vi "I-V measurement.vi"(5 "Session properties":T4, 7 "Workspace":path, 8 "Error In":errorcluster, 9 "myDLTS file path":path=path "", 10 "IV measurement":T1={"Name"="", "Comment"="", "Time"=timestamp(0 s since 1904-01-01), "Folder"=path "", "IV properties"={"T"=0.0, "Vstart"=-0.5, "Vstop"=0.5, "Vpoints"=10.0, "Settling"=0.01, "I limit"=0.1, "Log mapping"=FALSE, "Averaging"=0.0}, "GUID"=""} {"IV properties"."Settling" min=0.0 max=65535.0}, 11 "Loop data":T5={"Persistent"={"Last file"=path "", "Last user"="", "Users"=[]}, "Temp handle"={"Connected"=FALSE, "Temp ctrl"={"Gain (P)"=0.0, "Reset (I)"=0.0, "Rate (D)"=0.0, "Stabilization rate"=0.0, "Stabilization delta"=0.0, "Type"=enum."Lake Shore 325", "Custom temp ctrl"={"VISA resource name"=""}, "Lakeshore 325"={"VISA name"="", "Loop"=0, "Heater Range"=1, "Heater Resistance"=0, "Sample sensor"=0, "Fast sensor"=0, "Slow sensor"=0}, "Lakeshore 331"={"VISA name"="", "Loop"=1, "Heater Range"=0, "Sample sensor"=0, "Fast sensor"=0, "Slow sensor"=0}, "Lakeshore 332"={"VISA name"="", "Loop"=1, "Heater Range"=0, "Sample sensor"=0, "Fast sensor"=0, "Slow sensor"=0}, "Lakeshore 335"={"VISA name"="", "Loop"=1, "Sample sensor"=0, "Fast sensor"=0, "Slow sensor"=0, "Heater Range"=0, "Output mode"=enum."Off"}, "Lakeshore 336"={"VISA name"="", "Loop"=1, "Output mode"=enum."Off", "Max current"=1.0, "Heater resistance"=1, "Sample sensor"=1, "Slow sensor"=1, "Fast sensor"=1}}}, "Paths"={"Manual"=path "", "Settings"=path "", "Persistent"=path "", "Work dir."=path ""}, "Settings"={"MFIA"={"Address"="", "Use compensation"=TRUE, "Shut down gracefully"=FALSE}, "Temp ctrl"={"Gain (P)"=0.0, "Reset (I)"=0.0, "Rate (D)"=0.0, "Stabilization rate"=0.0, "Stabilization delta"=0.0, "Type"=enum."Lake Shore 325", "Custom temp ctrl"={"VISA resource name"=""}, "Lakeshore 325"={"VISA name"="", "Loop"=0, "Heater Range"=1, "Heater Resistance"=0, "Sample sensor"=0, "Fast sensor"=0, "Slow sensor"=0}, "Lakeshore 331"={"VISA name"="", "Loop"=1, "Heater Range"=0, "Sample sensor"=0, "Fast sensor"=0, "Slow sensor"=0}, "Lakeshore 332"={"VISA name"="", "Loop"=1, "Heater Range"=0, "Sample sensor"=0, "Fast sensor"=0, "Slow sensor"=0}, "Lakeshore 335"={"VISA name"="", "Loop"=1, "Sample sensor"=0, "Fast sensor"=0, "Slow sensor"=0, "Heater Range"=0, "Output mode"=enum."Off"}, "Lakeshore 336"={"VISA name"="", "Loop"=1, "Output mode"=enum."Off", "Max current"=1.0, "Heater resistance"=1, "Sample sensor"=1, "Slow sensor"=1, "Fast sensor"=1}}, "Source-meter"={"Type"=enum."Custom", "Custom source-meter"={"VISA resource name"=""}, "Keithley 2600"={"VISA name"="", "Ignore ID Query"=FALSE, "SMU"=enum."Channel A"}, "Keithley 2400 Series"={"VISA name"="", "Ignore ID Query"=FALSE}}, "Other"={"Enable OriginLab"=FALSE, "Reader mode"=FALSE, "Auto-save"=FALSE}, "Defaults"={"IV properties"={"T"=0.0, "Vstart"=-0.5, "Vstop"=0.5, "Vpoints"=10.0, "Settling"=0.01, "I limit"=0.1, "Log mapping"=FALSE, "Averaging"=0.0}, "CV properties"={"T"=0.0, "Vstart"=-0.5, "Vstop"=0.5, "Vpoints"=10.0, "Precision"=enum."Normal", "Test signal"=0.01, "Auto I range"=FALSE, "Test frequency"=100000.0, "I range"=-2.0, "V range"=10.0, "Log mapping"=FALSE, "Rel perm"=0.0, "Area"=0.0, "Equivalent circuit model"=0}, "DLTS properties"={"Tstart"=0.0, "Instant start"=FALSE, "Tstop"=0.0, "T rate"=0.0, "Test signal"=0.0, "Test frequency"=0.0, "Bandwidth"=0.0, "Averaging"=0.0, "Vbias"=0.0, "Vpulse"=0.0, "pulse length"=0.0, "Pulse 2"=FALSE, "Vpulse 2"=0.0, "pulse length 2"=0.0, "I range"=-2.0, "V range"=10.0, "Emission rate"=[], "Sampling rate"=0.0, "Acq. delay"=0.0, "Filter order"=0, "Equivalent circuit model"=0}, "LDLTS properties"={"T"=0.0, "Test signal"=0.0, "Test frequency"=0.0, "Bandwidth"=0.0, "Averaging"=0.0, "Vbias"=0.0, "Vpulse"=0.0, "pulse length"=0.0, "Pulse 2"=FALSE, "Vpulse 2"=0.0, "pulse length 2"=0.0, "I range"=-2.0, "V range"=10.0, "Sampling rate"=0.0, "Acq. delay"=0.0, "Sampling time"=0.0, "Filter order"=0, "Equivalent circuit model"=0}}}, "Software version"=0.0, "MFIA handle"={"ziHandle"={"handleValid"=FALSE, "Conn"=0, "Path Prefix"="", "Handle"=0, "Connected"=FALSE, "Clockbase(s)"=0.0}, "Selected device"="", "ziModHandle"={"handleValid"=FALSE, "Conn"=0, "ModHandle"=0, "moduleID"="", "Path Prefix"=""}}, "Source-meter handle"={"Connected"=FALSE, "Source-meter"={"Type"=enum."Custom", "Custom source-meter"={"VISA resource name"=""}, "Keithley 2600"={"VISA name"="", "Ignore ID Query"=FALSE, "SMU"=enum."Channel A"}, "Keithley 2400 Series"={"VISA name"="", "Ignore ID Query"=FALSE}}}} {"MFIA handle"."ziModHandle"."ModHandle" format="0x%08x"; "MFIA handle"."ziModHandle"."Conn" format="0x%08x"; "MFIA handle"."ziHandle"."Handle" format="0x%08x"; "MFIA handle"."ziHandle"."Conn" format="0x%08x"; "Settings"."Defaults"."LDLTS properties"."Equivalent circuit model" items=["Rp || Cp", "Rs + Cs", "Rs + Ls", "G B", "D Cs", "Q Cs", "D Ls", "Q Ls", "Rp || Lp", "D Cp"]; "Settings"."Defaults"."LDLTS properties"."Filter order" min=0 max=8 step=1; "Settings"."Defaults"."LDLTS properties"."Sampling rate" items=["13k"=13392.857422, "27k"=26785.714844, "54k"=53571.429687, "107k"=107142.859375]; "Settings"."Defaults"."LDLTS properties"."V range" items=["10mV"=0.01, "100mV"=0.1, "1V"=1.0, "10V"=10.0]; "Settings"."Defaults"."LDLTS properties"."I range" items=["100nA"=-7.0, "1µA"=-6.0, "10µA"=-5.0, "100µA"=-4.0, "1mA"=-3.0, "10mA"=-2.0]; "Settings"."Defaults"."DLTS properties"."Equivalent circuit model" items=["Rp || Cp", "Rs + Cs", "Rs + Ls", "G B", "D Cs", "Q Cs", "D Ls", "Q Ls", "Rp || Lp", "D Cp"]; "Settings"."Defaults"."DLTS properties"."Filter order" min=0 max=8 step=1; "Settings"."Defaults"."DLTS properties"."Sampling rate" items=["13k"=13392.857422, "27k"=26785.714844, "54k"=53571.429687, "107k"=107142.859375]; "Settings"."Defaults"."DLTS properties"."V range" items=["10mV"=0.01, "100mV"=0.1, "1V"=1.0, "10V"=10.0]; "Settings"."Defaults"."DLTS properties"."I range" items=["10mV"=0.01, "100mV"=0.1, "1V"=1.0, "10V"=10.0]; "Settings"."Defaults"."CV properties"."Equivalent circuit model" items=["Rp || Cp", "Rs + Cs", "Rs + Ls", "G B", "D Cs", "Q Cs", "D Ls", "Q Ls", "Rp || Lp", "D Cp"]; "Settings"."Defaults"."CV properties"."V range" items=["10mV"=0.01, "100mV"=0.1, "1V"=1.0, "10V"=10.0]; "Settings"."Defaults"."CV properties"."I range" items=["100nA"=-7.0, "1µA"=-6.0, "10µA"=-5.0, "100µA"=-4.0, "1mA"=-3.0, "10mA"=-2.0]; "Settings"."Defaults"."IV properties"."Settling" min=0.0 max=65535.0; "Settings"."Temp ctrl"."Lakeshore 336"."Fast sensor" items=["Sensor A", "Sensor B", "Sensor C", "Sensor D"]; "Settings"."Temp ctrl"."Lakeshore 336"."Slow sensor" items=["Sensor A", "Sensor B", "Sensor C", "Sensor D"]; "Settings"."Temp ctrl"."Lakeshore 336"."Sample sensor" items=["Sensor A", "Sensor B", "Sensor C", "Sensor D"]; "Settings"."Temp ctrl"."Lakeshore 336"."Heater resistance" items=["25 Ohm"=1, "50 Ohm"=2]; "Settings"."Temp ctrl"."Lakeshore 336"."Max current" items=["0.707 A"=0.0, "1 A"=1.0, "1.414 A"=1.414, "2 A"=2.0]; "Settings"."Temp ctrl"."Lakeshore 336"."Loop" items=["Output 1"=1, "Output 2"=2, "Output 3"=3, "Output 4"=4]; "Settings"."Temp ctrl"."Lakeshore 335"."Heater Range" items=["Off", "Low (On)", "Medium", "High"]; "Settings"."Temp ctrl"."Lakeshore 335"."Slow sensor" items=["A", "B"]; "Settings"."Temp ctrl"."Lakeshore 335"."Fast sensor" items=["A", "B"]; "Settings"."Temp ctrl"."Lakeshore 335"."Sample sensor" items=["A", "B"]; "Settings"."Temp ctrl"."Lakeshore 335"."Loop" items=["Loop 1"=1, "Loop 2"=2]; "Settings"."Temp ctrl"."Lakeshore 332"."Slow sensor" items=["A", "B"]; "Settings"."Temp ctrl"."Lakeshore 332"."Fast sensor" items=["A", "B"]; "Settings"."Temp ctrl"."Lakeshore 332"."Sample sensor" items=["A", "B"]; "Settings"."Temp ctrl"."Lakeshore 332"."Heater Range" items=["Off", "Low (0.5W)", "Med (5W)", "High (50W)"]; "Settings"."Temp ctrl"."Lakeshore 332"."Loop" items=["Loop 1", "Loop 2"]; "Settings"."Temp ctrl"."Lakeshore 331"."Slow sensor" items=["A", "B"]; "Settings"."Temp ctrl"."Lakeshore 331"."Fast sensor" items=["A", "B"]; "Settings"."Temp ctrl"."Lakeshore 331"."Sample sensor" items=["A", "B"]; "Settings"."Temp ctrl"."Lakeshore 331"."Heater Range" items=["Off", "Low (0.5W)", "Med (5W)", "High (50W)"]; "Settings"."Temp ctrl"."Lakeshore 331"."Loop" items=["Loop 1", "Loop 2"]; "Settings"."Temp ctrl"."Lakeshore 325"."Slow sensor" items=["A", "B"]; "Settings"."Temp ctrl"."Lakeshore 325"."Fast sensor" items=["A", "B"]; "Settings"."Temp ctrl"."Lakeshore 325"."Sample sensor" items=["A", "B"]; "Settings"."Temp ctrl"."Lakeshore 325"."Heater Resistance" items=["25 Ohm"=1, "50 Ohm"=2]; "Settings"."Temp ctrl"."Lakeshore 325"."Heater Range" items=["Off", "Low (loop 1) or On (loop 2)", "High (loop 1)"]; "Settings"."Temp ctrl"."Lakeshore 325"."Loop" items=["Loop 1"=1, "Loop 2"=2]; "Temp handle"."Temp ctrl"."Lakeshore 336"."Fast sensor" items=["Sensor A", "Sensor B", "Sensor C", "Sensor D"]; "Temp handle"."Temp ctrl"."Lakeshore 336"."Slow sensor" items=["Sensor A", "Sensor B", "Sensor C", "Sensor D"]; "Temp handle"."Temp ctrl"."Lakeshore 336"."Sample sensor" items=["Sensor A", "Sensor B", "Sensor C", "Sensor D"]; "Temp handle"."Temp ctrl"."Lakeshore 336"."Heater resistance" items=["25 Ohm"=1, "50 Ohm"=2]; "Temp handle"."Temp ctrl"."Lakeshore 336"."Max current" items=["0.707 A"=0.0, "1 A"=1.0, "1.414 A"=1.414, "2 A"=2.0]; "Temp handle"."Temp ctrl"."Lakeshore 336"."Loop" items=["Output 1"=1, "Output 2"=2, "Output 3"=3, "Output 4"=4]; "Temp handle"."Temp ctrl"."Lakeshore 335"."Heater Range" items=["Off", "Low (On)", "Medium", "High"]; "Temp handle"."Temp ctrl"."Lakeshore 335"."Slow sensor" items=["A", "B"]; "Temp handle"."Temp ctrl"."Lakeshore 335"."Fast sensor" items=["A", "B"]; "Temp handle"."Temp ctrl"."Lakeshore 335"."Sample sensor" items=["A", "B"]; "Temp handle"."Temp ctrl"."Lakeshore 335"."Loop" items=["Loop 1"=1, "Loop 2"=2]; "Temp handle"."Temp ctrl"."Lakeshore 332"."Slow sensor" items=["A", "B"]; "Temp handle"."Temp ctrl"."Lakeshore 332"."Fast sensor" items=["A", "B"]; "Temp handle"."Temp ctrl"."Lakeshore 332"."Sample sensor" items=["A", "B"]; "Temp handle"."Temp ctrl"."Lakeshore 332"."Heater Range" items=["Off", "Low (0.5W)", "Med (5W)", "High (50W)"]; "Temp handle"."Temp ctrl"."Lakeshore 332"."Loop" items=["Loop 1", "Loop 2"]; "Temp handle"."Temp ctrl"."Lakeshore 331"."Slow sensor" items=["A", "B"]; "Temp handle"."Temp ctrl"."Lakeshore 331"."Fast sensor" items=["A", "B"]; "Temp handle"."Temp ctrl"."Lakeshore 331"."Sample sensor" items=["A", "B"]; "Temp handle"."Temp ctrl"."Lakeshore 331"."Heater Range" items=["Off", "Low (0.5W)", "Med (5W)", "High (50W)"]; "Temp handle"."Temp ctrl"."Lakeshore 331"."Loop" items=["Loop 1", "Loop 2"]; "Temp handle"."Temp ctrl"."Lakeshore 325"."Slow sensor" items=["A", "B"]; "Temp handle"."Temp ctrl"."Lakeshore 325"."Fast sensor" items=["A", "B"]; "Temp handle"."Temp ctrl"."Lakeshore 325"."Sample sensor" items=["A", "B"]; "Temp handle"."Temp ctrl"."Lakeshore 325"."Heater Resistance" items=["25 Ohm"=1, "50 Ohm"=2]; "Temp handle"."Temp ctrl"."Lakeshore 325"."Heater Range" items=["Off", "Low (loop 1) or On (loop 2)", "High (loop 1)"]; "Temp handle"."Temp ctrl"."Lakeshore 325"."Loop" items=["Loop 1"=1, "Loop 2"=2]}) -> (0 "Error Out":errorcluster, 1 "Modified":bool, 2 "IV measurement out":T1={"Name"="", "Comment"="", "Time"=timestamp(0 s since 1904-01-01), "Folder"=path "", "IV properties"={"T"=0.0, "Vstart"=-0.5, "Vstop"=0.5, "Vpoints"=10.0, "Settling"=0.01, "I limit"=0.1, "Log mapping"=FALSE, "Averaging"=0.0}, "GUID"=""} {"IV properties"."Settling" min=0.0 max=65535.0}, 3 "Loop data out":T5={"Persistent"={"Last file"=path "", "Last user"="", "Users"=[]}, "Temp handle"={"Connected"=FALSE, "Temp ctrl"={"Gain (P)"=0.0, "Reset (I)"=0.0, "Rate (D)"=0.0, "Stabilization rate"=0.0, "Stabilization delta"=0.0, "Type"=enum."Lake Shore 325", "Custom temp ctrl"={"VISA resource name"=""}, "Lakeshore 325"={"VISA name"="", "Loop"=0, "Heater Range"=1, "Heater Resistance"=0, "Sample sensor"=0, "Fast sensor"=0, "Slow sensor"=0}, "Lakeshore 331"={"VISA name"="", "Loop"=1, "Heater Range"=0, "Sample sensor"=0, "Fast sensor"=0, "Slow sensor"=0}, "Lakeshore 332"={"VISA name"="", "Loop"=1, "Heater Range"=0, "Sample sensor"=0, "Fast sensor"=0, "Slow sensor"=0}, "Lakeshore 335"={"VISA name"="", "Loop"=1, "Sample sensor"=0, "Fast sensor"=0, "Slow sensor"=0, "Heater Range"=0, "Output mode"=enum."Off"}, "Lakeshore 336"={"VISA name"="", "Loop"=1, "Output mode"=enum."Off", "Max current"=1.0, "Heater resistance"=1, "Sample sensor"=1, "Slow sensor"=1, "Fast sensor"=1}}}, "Paths"={"Manual"=path "", "Settings"=path "", "Persistent"=path "", "Work dir."=path ""}, "Settings"={"MFIA"={"Address"="", "Use compensation"=TRUE, "Shut down gracefully"=FALSE}, "Temp ctrl"={"Gain (P)"=0.0, "Reset (I)"=0.0, "Rate (D)"=0.0, "Stabilization rate"=0.0, "Stabilization delta"=0.0, "Type"=enum."Lake Shore 325", "Custom temp ctrl"={"VISA resource name"=""}, "Lakeshore 325"={"VISA name"="", "Loop"=0, "Heater Range"=1, "Heater Resistance"=0, "Sample sensor"=0, "Fast sensor"=0, "Slow sensor"=0}, "Lakeshore 331"={"VISA name"="", "Loop"=1, "Heater Range"=0, "Sample sensor"=0, "Fast sensor"=0, "Slow sensor"=0}, "Lakeshore 332"={"VISA name"="", "Loop"=1, "Heater Range"=0, "Sample sensor"=0, "Fast sensor"=0, "Slow sensor"=0}, "Lakeshore 335"={"VISA name"="", "Loop"=1, "Sample sensor"=0, "Fast sensor"=0, "Slow sensor"=0, "Heater Range"=0, "Output mode"=enum."Off"}, "Lakeshore 336"={"VISA name"="", "Loop"=1, "Output mode"=enum."Off", "Max current"=1.0, "Heater resistance"=1, "Sample sensor"=1, "Slow sensor"=1, "Fast sensor"=1}}, "Source-meter"={"Type"=enum."Custom", "Custom source-meter"={"VISA resource name"=""}, "Keithley 2600"={"VISA name"="", "Ignore ID Query"=FALSE, "SMU"=enum."Channel A"}, "Keithley 2400 Series"={"VISA name"="", "Ignore ID Query"=FALSE}}, "Other"={"Enable OriginLab"=FALSE, "Reader mode"=FALSE, "Auto-save"=FALSE}, "Defaults"={"IV properties"={"T"=0.0, "Vstart"=-0.5, "Vstop"=0.5, "Vpoints"=10.0, "Settling"=0.01, "I limit"=0.1, "Log mapping"=FALSE, "Averaging"=0.0}, "CV properties"={"T"=0.0, "Vstart"=-0.5, "Vstop"=0.5, "Vpoints"=10.0, "Precision"=enum."Normal", "Test signal"=0.01, "Auto I range"=FALSE, "Test frequency"=100000.0, "I range"=-2.0, "V range"=10.0, "Log mapping"=FALSE, "Rel perm"=0.0, "Area"=0.0, "Equivalent circuit model"=0}, "DLTS properties"={"Tstart"=0.0, "Instant start"=FALSE, "Tstop"=0.0, "T rate"=0.0, "Test signal"=0.0, "Test frequency"=0.0, "Bandwidth"=0.0, "Averaging"=0.0, "Vbias"=0.0, "Vpulse"=0.0, "pulse length"=0.0, "Pulse 2"=FALSE, "Vpulse 2"=0.0, "pulse length 2"=0.0, "I range"=-2.0, "V range"=10.0, "Emission rate"=[], "Sampling rate"=0.0, "Acq. delay"=0.0, "Filter order"=0, "Equivalent circuit model"=0}, "LDLTS properties"={"T"=0.0, "Test signal"=0.0, "Test frequency"=0.0, "Bandwidth"=0.0, "Averaging"=0.0, "Vbias"=0.0, "Vpulse"=0.0, "pulse length"=0.0, "Pulse 2"=FALSE, "Vpulse 2"=0.0, "pulse length 2"=0.0, "I range"=-2.0, "V range"=10.0, "Sampling rate"=0.0, "Acq. delay"=0.0, "Sampling time"=0.0, "Filter order"=0, "Equivalent circuit model"=0}}}, "Software version"=0.0, "MFIA handle"={"ziHandle"={"handleValid"=FALSE, "Conn"=0, "Path Prefix"="", "Handle"=0, "Connected"=FALSE, "Clockbase(s)"=0.0}, "Selected device"="", "ziModHandle"={"handleValid"=FALSE, "Conn"=0, "ModHandle"=0, "moduleID"="", "Path Prefix"=""}}, "Source-meter handle"={"Connected"=FALSE, "Source-meter"={"Type"=enum."Custom", "Custom source-meter"={"VISA resource name"=""}, "Keithley 2600"={"VISA name"="", "Ignore ID Query"=FALSE, "SMU"=enum."Channel A"}, "Keithley 2400 Series"={"VISA name"="", "Ignore ID Query"=FALSE}}}} {"MFIA handle"."ziModHandle"."ModHandle" format="0x%08x"; "MFIA handle"."ziModHandle"."Conn" format="0x%08x"; "MFIA handle"."ziHandle"."Handle" format="0x%08x"; "MFIA handle"."ziHandle"."Conn" format="0x%08x"; "Settings"."Defaults"."LDLTS properties"."Equivalent circuit model" items=["Rp || Cp", "Rs + Cs", "Rs + Ls", "G B", "D Cs", "Q Cs", "D Ls", "Q Ls", "Rp || Lp", "D Cp"]; "Settings"."Defaults"."LDLTS properties"."Filter order" min=0 max=8 step=1; "Settings"."Defaults"."LDLTS properties"."Sampling rate" items=["13k"=13392.857422, "27k"=26785.714844, "54k"=53571.429687, "107k"=107142.859375]; "Settings"."Defaults"."LDLTS properties"."V range" items=["10mV"=0.01, "100mV"=0.1, "1V"=1.0, "10V"=10.0]; "Settings"."Defaults"."LDLTS properties"."I range" items=["100nA"=-7.0, "1µA"=-6.0, "10µA"=-5.0, "100µA"=-4.0, "1mA"=-3.0, "10mA"=-2.0]; "Settings"."Defaults"."DLTS properties"."Equivalent circuit model" items=["Rp || Cp", "Rs + Cs", "Rs + Ls", "G B", "D Cs", "Q Cs", "D Ls", "Q Ls", "Rp || Lp", "D Cp"]; "Settings"."Defaults"."DLTS properties"."Filter order" min=0 max=8 step=1; "Settings"."Defaults"."DLTS properties"."Sampling rate" items=["13k"=13392.857422, "27k"=26785.714844, "54k"=53571.429687, "107k"=107142.859375]; "Settings"."Defaults"."DLTS properties"."V range" items=["10mV"=0.01, "100mV"=0.1, "1V"=1.0, "10V"=10.0]; "Settings"."Defaults"."DLTS properties"."I range" items=["10mV"=0.01, "100mV"=0.1, "1V"=1.0, "10V"=10.0]; "Settings"."Defaults"."CV properties"."Equivalent circuit model" items=["Rp || Cp", "Rs + Cs", "Rs + Ls", "G B", "D Cs", "Q Cs", "D Ls", "Q Ls", "Rp || Lp", "D Cp"]; "Settings"."Defaults"."CV properties"."V range" items=["10mV"=0.01, "100mV"=0.1, "1V"=1.0, "10V"=10.0]; "Settings"."Defaults"."CV properties"."I range" items=["100nA"=-7.0, "1µA"=-6.0, "10µA"=-5.0, "100µA"=-4.0, "1mA"=-3.0, "10mA"=-2.0]; "Settings"."Defaults"."IV properties"."Settling" min=0.0 max=65535.0; "Settings"."Temp ctrl"."Lakeshore 336"."Fast sensor" items=["Sensor A", "Sensor B", "Sensor C", "Sensor D"]; "Settings"."Temp ctrl"."Lakeshore 336"."Slow sensor" items=["Sensor A", "Sensor B", "Sensor C", "Sensor D"]; "Settings"."Temp ctrl"."Lakeshore 336"."Sample sensor" items=["Sensor A", "Sensor B", "Sensor C", "Sensor D"]; "Settings"."Temp ctrl"."Lakeshore 336"."Heater resistance" items=["25 Ohm"=1, "50 Ohm"=2]; "Settings"."Temp ctrl"."Lakeshore 336"."Max current" items=["0.707 A"=0.0, "1 A"=1.0, "1.414 A"=1.414, "2 A"=2.0]; "Settings"."Temp ctrl"."Lakeshore 336"."Loop" items=["Output 1"=1, "Output 2"=2, "Output 3"=3, "Output 4"=4]; "Settings"."Temp ctrl"."Lakeshore 335"."Heater Range" items=["Off", "Low (On)", "Medium", "High"]; "Settings"."Temp ctrl"."Lakeshore 335"."Slow sensor" items=["A", "B"]; "Settings"."Temp ctrl"."Lakeshore 335"."Fast sensor" items=["A", "B"]; "Settings"."Temp ctrl"."Lakeshore 335"."Sample sensor" items=["A", "B"]; "Settings"."Temp ctrl"."Lakeshore 335"."Loop" items=["Loop 1"=1, "Loop 2"=2]; "Settings"."Temp ctrl"."Lakeshore 332"."Slow sensor" items=["A", "B"]; "Settings"."Temp ctrl"."Lakeshore 332"."Fast sensor" items=["A", "B"]; "Settings"."Temp ctrl"."Lakeshore 332"."Sample sensor" items=["A", "B"]; "Settings"."Temp ctrl"."Lakeshore 332"."Heater Range" items=["Off", "Low (0.5W)", "Med (5W)", "High (50W)"]; "Settings"."Temp ctrl"."Lakeshore 332"."Loop" items=["Loop 1", "Loop 2"]; "Settings"."Temp ctrl"."Lakeshore 331"."Slow sensor" items=["A", "B"]; "Settings"."Temp ctrl"."Lakeshore 331"."Fast sensor" items=["A", "B"]; "Settings"."Temp ctrl"."Lakeshore 331"."Sample sensor" items=["A", "B"]; "Settings"."Temp ctrl"."Lakeshore 331"."Heater Range" items=["Off", "Low (0.5W)", "Med (5W)", "High (50W)"]; "Settings"."Temp ctrl"."Lakeshore 331"."Loop" items=["Loop 1", "Loop 2"]; "Settings"."Temp ctrl"."Lakeshore 325"."Slow sensor" items=["A", "B"]; "Settings"."Temp ctrl"."Lakeshore 325"."Fast sensor" items=["A", "B"]; "Settings"."Temp ctrl"."Lakeshore 325"."Sample sensor" items=["A", "B"]; "Settings"."Temp ctrl"."Lakeshore 325"."Heater Resistance" items=["25 Ohm"=1, "50 Ohm"=2]; "Settings"."Temp ctrl"."Lakeshore 325"."Heater Range" items=["Off", "Low (loop 1) or On (loop 2)", "High (loop 1)"]; "Settings"."Temp ctrl"."Lakeshore 325"."Loop" items=["Loop 1"=1, "Loop 2"=2]; "Temp handle"."Temp ctrl"."Lakeshore 336"."Fast sensor" items=["Sensor A", "Sensor B", "Sensor C", "Sensor D"]; "Temp handle"."Temp ctrl"."Lakeshore 336"."Slow sensor" items=["Sensor A", "Sensor B", "Sensor C", "Sensor D"]; "Temp handle"."Temp ctrl"."Lakeshore 336"."Sample sensor" items=["Sensor A", "Sensor B", "Sensor C", "Sensor D"]; "Temp handle"."Temp ctrl"."Lakeshore 336"."Heater resistance" items=["25 Ohm"=1, "50 Ohm"=2]; "Temp handle"."Temp ctrl"."Lakeshore 336"."Max current" items=["0.707 A"=0.0, "1 A"=1.0, "1.414 A"=1.414, "2 A"=2.0]; "Temp handle"."Temp ctrl"."Lakeshore 336"."Loop" items=["Output 1"=1, "Output 2"=2, "Output 3"=3, "Output 4"=4]; "Temp handle"."Temp ctrl"."Lakeshore 335"."Heater Range" items=["Off", "Low (On)", "Medium", "High"]; "Temp handle"."Temp ctrl"."Lakeshore 335"."Slow sensor" items=["A", "B"]; "Temp handle"."Temp ctrl"."Lakeshore 335"."Fast sensor" items=["A", "B"]; "Temp handle"."Temp ctrl"."Lakeshore 335"."Sample sensor" items=["A", "B"]; "Temp handle"."Temp ctrl"."Lakeshore 335"."Loop" items=["Loop 1"=1, "Loop 2"=2]; "Temp handle"."Temp ctrl"."Lakeshore 332"."Slow sensor" items=["A", "B"]; "Temp handle"."Temp ctrl"."Lakeshore 332"."Fast sensor" items=["A", "B"]; "Temp handle"."Temp ctrl"."Lakeshore 332"."Sample sensor" items=["A", "B"]; "Temp handle"."Temp ctrl"."Lakeshore 332"."Heater Range" items=["Off", "Low (0.5W)", "Med (5W)", "High (50W)"]; "Temp handle"."Temp ctrl"."Lakeshore 332"."Loop" items=["Loop 1", "Loop 2"]; "Temp handle"."Temp ctrl"."Lakeshore 331"."Slow sensor" items=["A", "B"]; "Temp handle"."Temp ctrl"."Lakeshore 331"."Fast sensor" items=["A", "B"]; "Temp handle"."Temp ctrl"."Lakeshore 331"."Sample sensor" items=["A", "B"]; "Temp handle"."Temp ctrl"."Lakeshore 331"."Heater Range" items=["Off", "Low (0.5W)", "Med (5W)", "High (50W)"]; "Temp handle"."Temp ctrl"."Lakeshore 331"."Loop" items=["Loop 1", "Loop 2"]; "Temp handle"."Temp ctrl"."Lakeshore 325"."Slow sensor" items=["A", "B"]; "Temp handle"."Temp ctrl"."Lakeshore 325"."Fast sensor" items=["A", "B"]; "Temp handle"."Temp ctrl"."Lakeshore 325"."Sample sensor" items=["A", "B"]; "Temp handle"."Temp ctrl"."Lakeshore 325"."Heater Resistance" items=["25 Ohm"=1, "50 Ohm"=2]; "Temp handle"."Temp ctrl"."Lakeshore 325"."Heater Range" items=["Off", "Low (loop 1) or On (loop 2)", "High (loop 1)"]; "Temp handle"."Temp ctrl"."Lakeshore 325"."Loop" items=["Loop 1"=1, "Loop 2"=2]})   [LabVIEW 2019]
doc: "Handles I-V measurement, displays I-V GUI window"
uses:
  Type defs/Loop data Type Def.ctl
  Type defs/Persistent Type Def.ctl
  Type defs/Temp handle Type Def.ctl
  Type defs/Temp ctrl Type Def.ctl
  Custom devices/Custom temp ctrl settings.ctl
  Type defs/Paths Type Def.ctl
  Type defs/Settings Type Def.ctl
  Type defs/Imps Type Def.ctl
  Type defs/Source-meter Type Def.ctl
  Custom devices/Custom source-meter settings.ctl
  Type defs/Other settings Type Def.ctl
  Type defs/IV properties Type Def.ctl
  Type defs/CV properties Type Def.ctl
  Type defs/DLTS properties Type Def.ctl
  Type defs/LDLTS properties Type Def.ctl
  Type defs/MFIA handle Type Def.ctl
  <instrlib>/Zurich Instruments LabOne/Public/ziTypeHandle.ctl
  <instrlib>/Zurich Instruments LabOne/Public/Modules/ziTypeModHandle.ctl
  Type defs/Source-meter handle Type Def.ctl
  Type defs/Session properties Type Def.ctl
  Type defs/IV measurement Type Def.ctl
  <vilib>/Utility/error.llb/DialogType.ctl
  <vilib>/TaskbarProgressAPI/_TypeDefs/Progress State.ctl
  510f3f78-f7bb-479b-aecc-521aa5b5f88d.vi
  Export single dat - IV cluster.vi
  Export single clipboard - IV cluster.vi
  Export Origin - IV.vi
  <vilib>/TaskbarProgressAPI/TaskbarProgressAPI.lvlib
  <instrlib>/Zurich Instruments LabOne/Zurich Instruments LabOne.lvlib
panel:
  in  "Stop":bool
  in  "Folder":path
  in  "Swap V":bool
  out "Voltage step":dbl[unit]=-0.5 caption="Numeric" format="%#_6p"
  in  "Averaging":dbl=1.0 caption="Numeric" min=1.0 max=100.0 step=1.0 format="%#_6p"
  in  "Semi-log graph display":bool
  in  "Settling":dbl[unit] caption="Numeric" min=0.0 format="%#_6p"
  in  "Buttons":T3
  in  "Log mapping":bool caption="Log dist."
  out "Measurement info":string
  in  "Current limit":dbl[unit]=100.0 caption="Numeric" format="%#_6p"
  in  "Measure":bool
  in  "Voltage points":dbl=100.0 caption="Numeric" min=2.0 max=2001.0 step=1.0
  in  "End voltage":dbl[unit]=0.5 caption="Numeric" format="%#_6p"
  in  "Start voltage":dbl[unit]=-0.5 caption="Numeric" format="%#_6p"
  in  "Setpoint":dbl[unit]=1.0 caption="Numeric" min=1.0 max=800.0
  out "Temperature":dbl[unit] caption="Numeric"
  in  "Connect":bool
  out "I-V":cluster{"2D data":dbl[], "2D data":dbl[]}(graph)
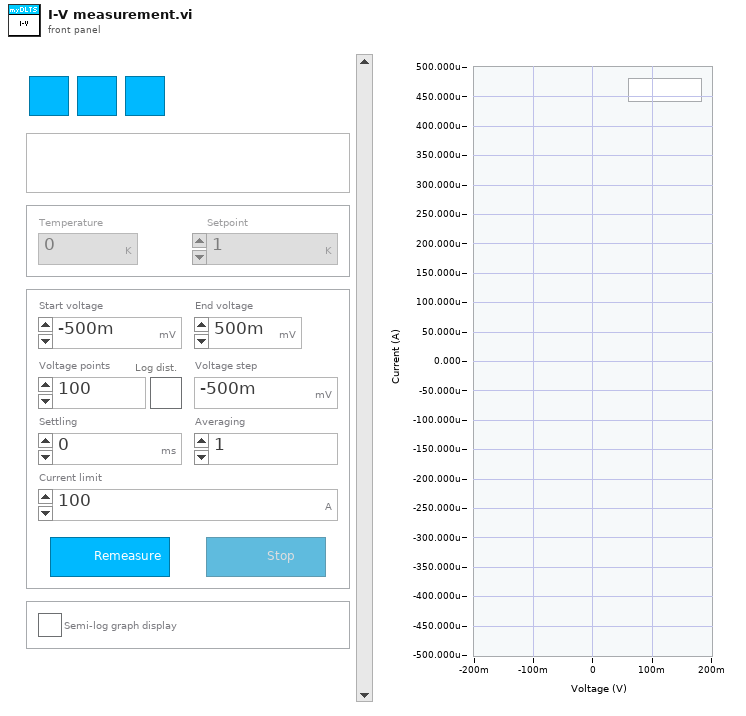
[diagram p1: front panel]
types:
  T1 = typedef "IV measurement Type Def.ctl" = cluster{"Name":string, "Comment":string, "Time":timestamp, "Folder":path, "IV properties":T2, "GUID":string}
  T2 = typedef "IV properties Type Def.ctl" = cluster{"T":dbl[unit], "Vstart":dbl[unit], "Vstop":dbl[unit], "Vpoints":dbl, "Settling":dbl[unit], "I limit":dbl[unit], "Log mapping":bool, "Averaging":dbl}
  T3 = cluster{"Information":bool, "Help":bool, "Export":bool}
  T4 = typedef "Session properties Type Def.ctl" = cluster{"Session name":string, "Comment":string, "User":string, "Software version":dbl, "Created":timestamp, "Modified":timestamp, "Binary":bool, "GUID":string}
  T5 = typedef "Loop data Type Def.ctl" = cluster{"Persistent":T6, "Temp handle":T7, "Paths":T10, "Settings":T11, "Software version":dbl, "MFIA handle":T19, "Source-meter handle":T22}
  T6 = typedef "Persistent Type Def.ctl" = cluster{"Last file":path, "Last user":string, "Users":cluster{"User":string, "Authors directory":path}[]}
  T7 = typedef "Temp handle Type Def.ctl" = cluster{"Connected":bool, "Temp ctrl":T8}
  T8 = typedef "Temp ctrl Type Def.ctl" = cluster{"Gain (P)":dbl, "Reset (I)":dbl, "Rate (D)":dbl, "Stabilization rate":dbl, "Stabilization delta":dbl, "Type":enum16{"Custom", "Lake Shore 325", "Lake Shore 331", "Lake Shore 332", "Lake Shore 335", "Lake Shore 336"}, "Custom temp ctrl":T9, "Lakeshore 325":cluster{"VISA name":refnum<visa-resource-name>, "Loop":u16, "Heater Range":u16, "Heater Resistance":u16, "Sample sensor":u16, "Fast sensor":u16, "Slow sensor":u16}, "Lakeshore 331":cluster{"VISA name":refnum<visa-resource-name>, "Loop":u16, "Heater Range":u16, "Sample sensor":u16, "Fast sensor":u16, "Slow sensor":u16}, "Lakeshore 332":cluster{"VISA name":refnum<visa-resource-name>, "Loop":u16, "Heater Range":u16, "Sample sensor":u16, "Fast sensor":u16, "Slow sensor":u16}, "Lakeshore 335":cluster{"VISA name":refnum<visa-resource-name>, "Loop":u16, "Sample sensor":u16, "Fast sensor":u16, "Slow sensor":u16, "Heater Range":u16, "Output mode":enum16{"Off", "Closed Loop PID", "Zone", "Open Loop", "Monitor Out", "Warmup Supply"}}, "Lakeshore 336":cluster{"VISA name":refnum<visa-resource-name>, "Loop":u16, "Output mode":enum16{"Off", "Closed Loop PID", "Zone", "Open Loop"}, "Max current":dbl, "Heater resistance":u16, "Sample sensor":u16, "Slow sensor":u16, "Fast sensor":u16}}
  T9 = typedef "Custom temp ctrl settings.ctl" = cluster{"VISA resource name":refnum<visa-resource-name>}
  T10 = typedef "Paths Type Def.ctl" = cluster{"Manual":path, "Settings":path, "Persistent":path, "Work dir.":path}
  T11 = typedef "Settings Type Def.ctl" = cluster{"MFIA":T12, "Temp ctrl":T8, "Source-meter":T13, "Other":T15, "Defaults":cluster{"IV properties":T2, "CV properties":T16, "DLTS properties":T17, "LDLTS properties":T18}}
  T12 = typedef "Imps Type Def.ctl" = cluster{"Address":string, "Use compensation":bool, "Shut down gracefully":bool}
  T13 = typedef "Source-meter Type Def.ctl" = cluster{"Type":enum16{"Custom", "Keithley 2600", "Keithley 2400 Series"}, "Custom source-meter":T14, "Keithley 2600":cluster{"VISA name":refnum<visa-resource-name>, "Ignore ID Query":bool, "SMU":enum16{"Channel A", "Channel B"}}, "Keithley 2400 Series":cluster{"VISA name":refnum<visa-resource-name>, "Ignore ID Query":bool}}
  T14 = typedef "Custom source-meter settings.ctl" = cluster{"VISA resource name":refnum<visa-resource-name>}
  T15 = typedef "Other settings Type Def.ctl" = cluster{"Enable OriginLab":bool, "Reader mode":bool, "Auto-save":bool}
  T16 = typedef "CV properties Type Def.ctl" = cluster{"T":dbl[unit], "Vstart":dbl[unit], "Vstop":dbl[unit], "Vpoints":dbl, "Precision":enum16{"Low (Fast)", "Normal", "High (Slow)"}, "Test signal":dbl[unit], "Auto I range":bool, "Test frequency":dbl[unit], "I range":dbl, "V range":dbl[unit], "Log mapping":bool, "Rel perm":dbl, "Area":dbl[unit], "Equivalent circuit model":u16}
  T17 = typedef "DLTS properties Type Def.ctl" = cluster{"Tstart":dbl[unit], "Instant start":bool, "Tstop":dbl[unit], "T rate":dbl[unit], "Test signal":dbl[unit], "Test frequency":dbl[unit], "Bandwidth":dbl[unit], "Averaging":dbl, "Vbias":dbl[unit], "Vpulse":dbl[unit], "pulse length":dbl[unit], "Pulse 2":bool, "Vpulse 2":dbl[unit], "pulse length 2":dbl[unit], "I range":dbl, "V range":dbl[unit], "Emission rate":dbl[unit][], "Sampling rate":dbl[unit], "Acq. delay":dbl[unit], "Filter order":i32, "Equivalent circuit model":u16}
  T18 = typedef "LDLTS properties Type Def.ctl" = cluster{"T":dbl[unit], "Test signal":dbl[unit], "Test frequency":dbl[unit], "Bandwidth":dbl[unit], "Averaging":dbl, "Vbias":dbl[unit], "Vpulse":dbl[unit], "pulse length":dbl[unit], "Pulse 2":bool, "Vpulse 2":dbl[unit], "pulse length 2":dbl[unit], "I range":dbl, "V range":dbl[unit], "Sampling rate":dbl[unit], "Acq. delay":dbl[unit], "Sampling time":dbl[unit], "Filter order":i32, "Equivalent circuit model":u16}
  T19 = typedef "MFIA handle Type Def.ctl" = cluster{"ziHandle":T20, "Selected device":string, "ziModHandle":T21}
  T20 = typedef "Zurich Instruments LabOne.lvlib/ziTypeHandle.ctl" = cluster{"handleValid":bool, "Conn":u64, "Path Prefix":string, "Handle":u64, "Connected":bool, "Clockbase(s)":dbl}
  T21 = typedef "Zurich Instruments LabOne.lvlib/ziTypeModHandle.ctl" = cluster{"handleValid":bool, "Conn":u64, "ModHandle":u64, "moduleID":string, "Path Prefix":string}
  T22 = typedef "Source-meter handle Type Def.ctl" = cluster{"Connected":bool, "Source-meter":T13}
  T23 = enum8{"Enabled", "Disabled", "Disabled and Grayed Out"}
  T24 = cluster{"MFIA":bool, "Temperature controller":bool, "Source meter":bool}
  T25 = enum8{"Decimal", "Scientific", "Engineering", "Binary", "Octal", "Hexadecimal", "Relative time", "Time and date", "SI"}
  T26 = cluster{"Clipboard":bool, "dat":bool, "iso":bool, "Origin":bool, "Excel":bool}
  T27 = typedef "DialogType.ctl" = u16
  T28 = enum16{"Canceled", "Clipboard", "Dat", "Iso", "Origin", "Excel"}
  T29 = typedef "TaskbarProgressAPI.lvlib/Progress State.ctl" = i32
  T30 = cluster{"Voltage (V)":dbl[], "Current (A)":dbl[]}
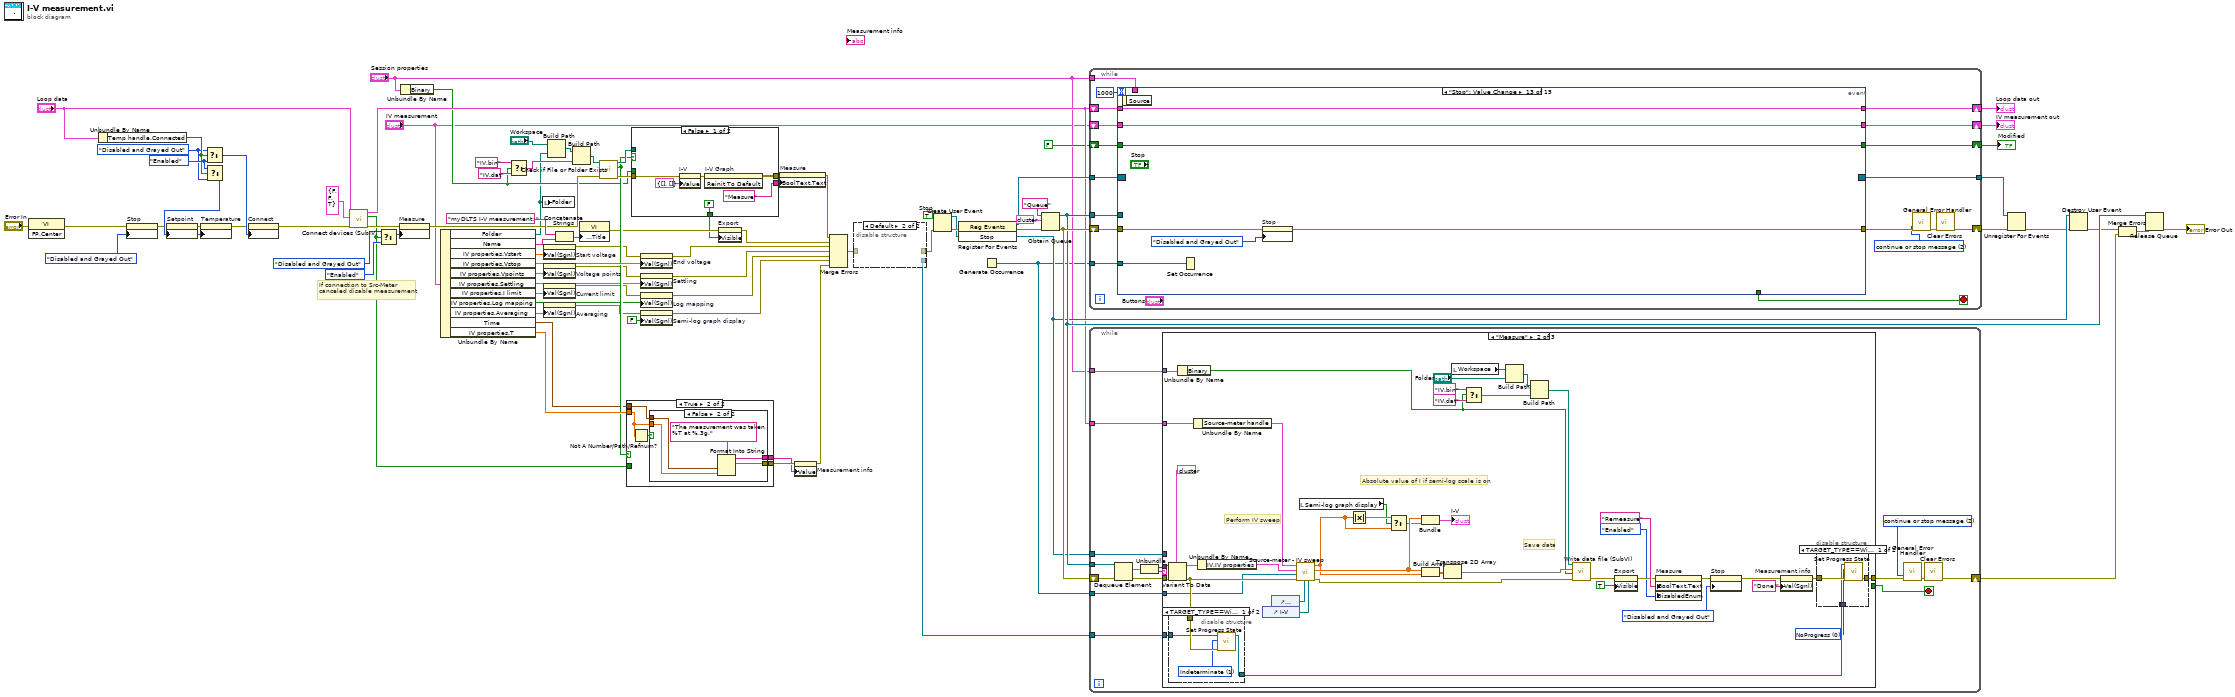
[diagram p0: block diagram]
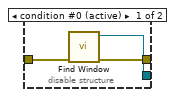
[diagram p2: hidden frame]
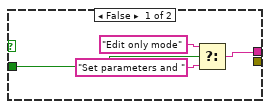
[diagram p3: hidden frame]
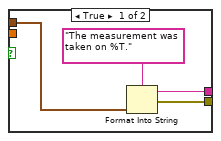
[diagram p4: hidden frame]
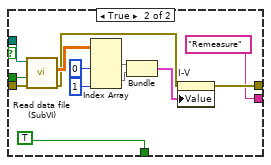
[diagram p5: hidden frame]
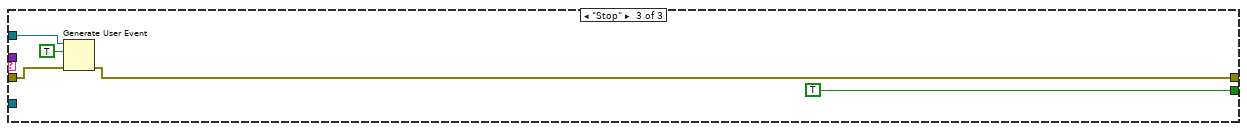
[diagram p9: hidden frame]
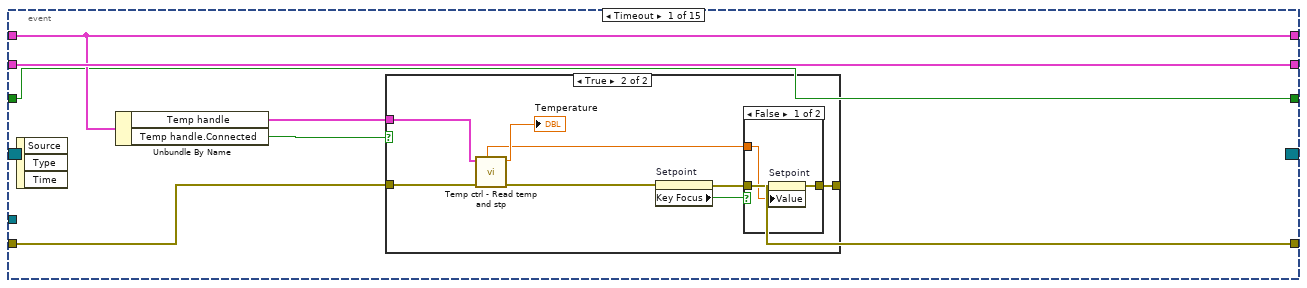
[diagram p10: hidden frame]
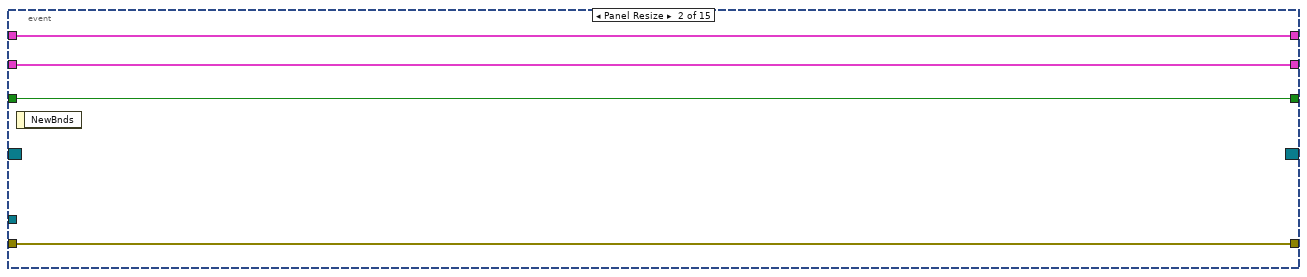
[diagram p13: hidden frame]
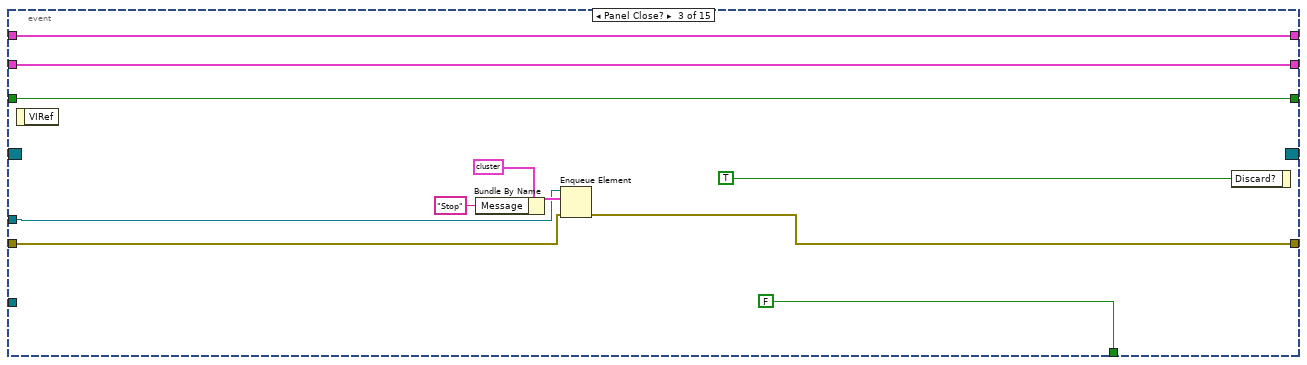
[diagram p14: hidden frame]
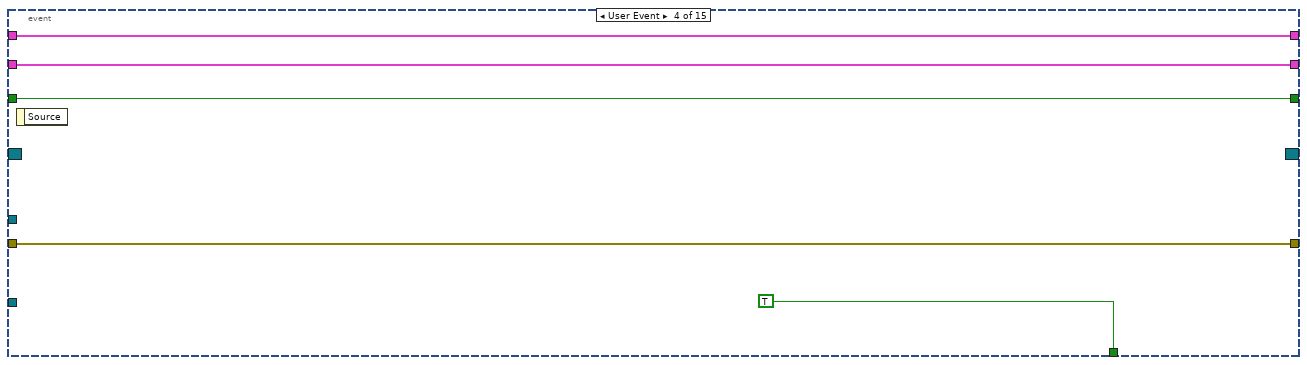
[diagram p15: hidden frame]
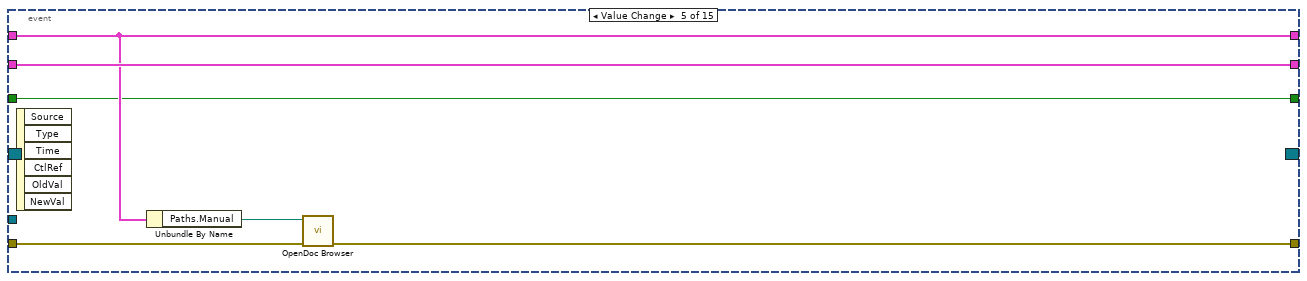
[diagram p16: hidden frame]
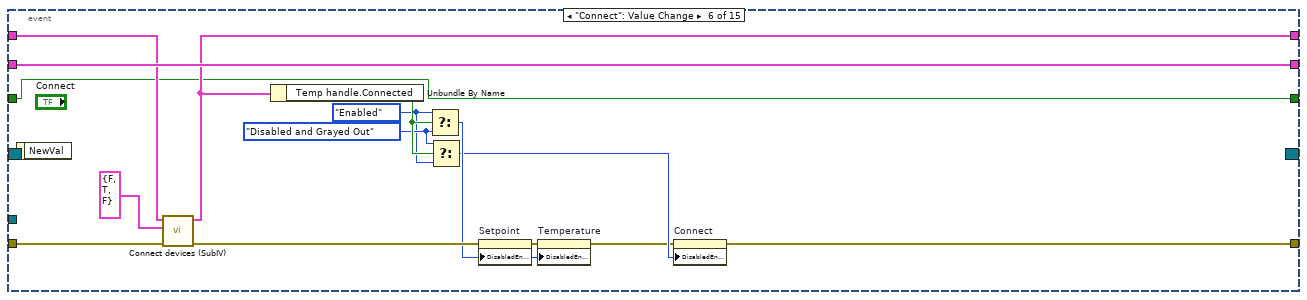
[diagram p17: hidden frame]
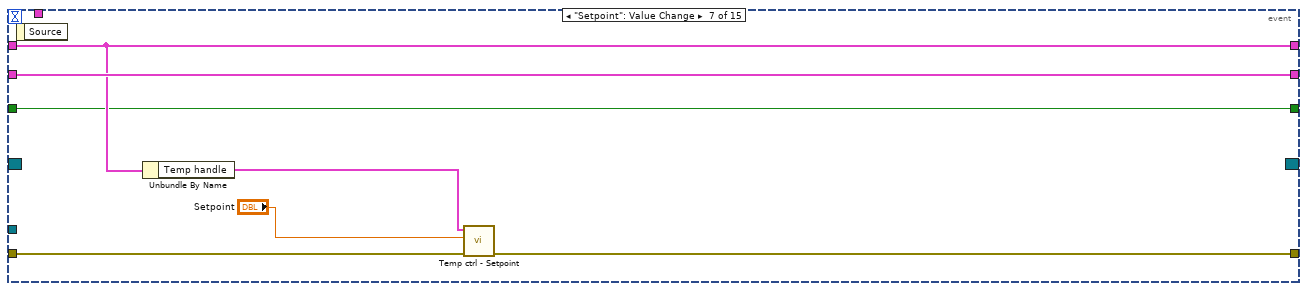
[diagram p18: hidden frame]
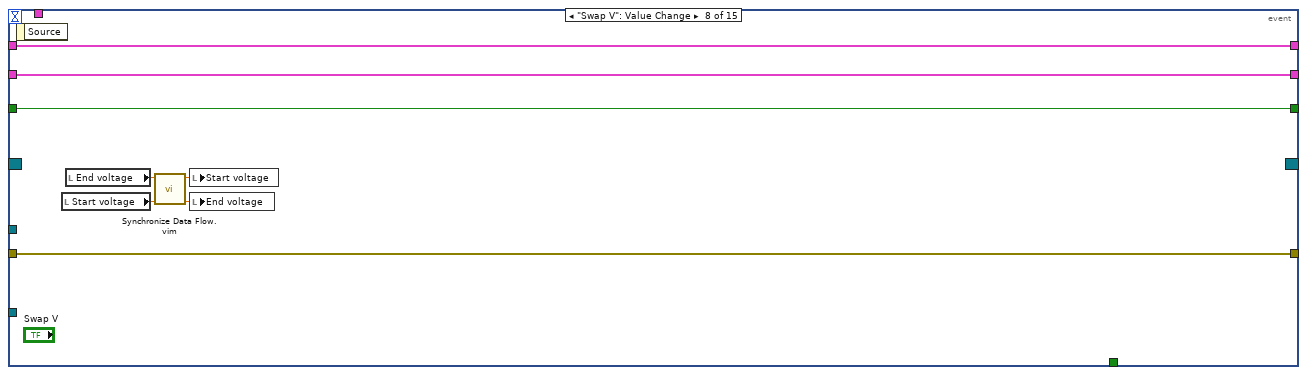
[diagram p19: hidden frame]
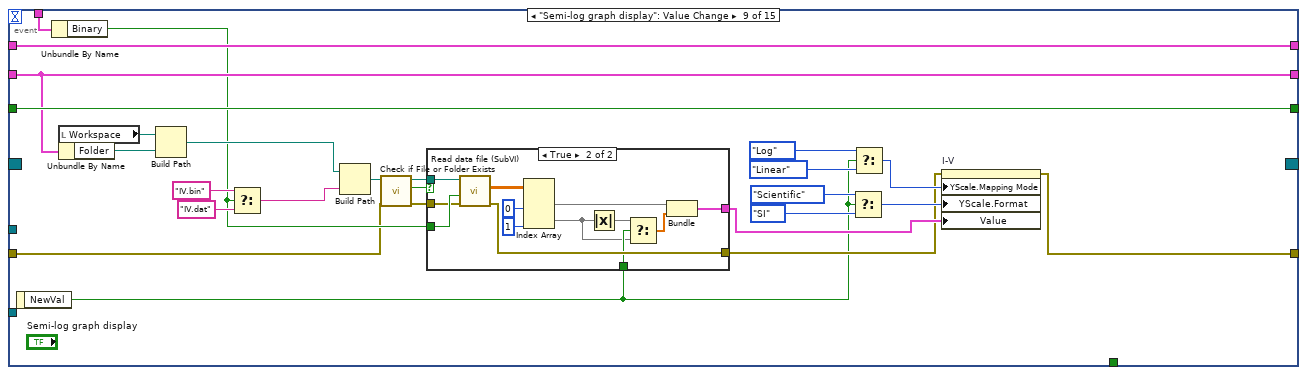
[diagram p20: hidden frame]
diagram:
  w68 = TRUE  # Stop
  w85 = T23."Enabled" ("f")
  w84 = T23."Disabled and Grayed Out" ("Disabled")
  # "If connection to Src-Meter canceled disable measurement"
  n1 = invoke class="VI" method="FP.Center"(error in="Error In") -> (error out=w4:errorcluster)  [unwired: 2 in, 2 out]
  n2 = Unbundle By Name("Loop data") -> ("Temp handle.Connected"=w86:bool)
  n3 = property on="Stop" class="Bool"(error in=w4, "DisabledEnum"=T23."Disabled and Grayed Out" ("Disabled")) -> (error out=w3:errorcluster)  [unwired: 1 in, 1 out]
  n4 = Select(t=w84, s=w86, f=w85) -> (s? t:f=w67:T23)
  n5 = Select(t=w85, s=w86, f=w84) -> (s? t:f=w66:T23)
  n6 = property on="Setpoint" class="DigNum (strict)"(error in=w3, "DisabledEnum"=w66) -> (error out=w87:errorcluster)  [unwired: 1 in, 1 out]
  n7 = property on="Temperature" class="DigNum (strict)"(error in=w87, "DisabledEnum"=w66) -> (error out=w22:errorcluster)  [unwired: 1 in, 1 out]
  n8 = property on="Connect" class="Bool"(error in=w22, "DisabledEnum"=w67) -> (error out=w47:errorcluster)  [unwired: 1 in, 1 out]
  n9 = call "Connect devices (SubIV).vi"("Error In"=w47, "Devices"=T24 {"MFIA"=FALSE, "Temperature controller"=FALSE, "Source meter"=TRUE}, "Loop data in"="Loop data") -> ("Error Out"=w83:errorcluster, "Canceled"=w53:bool, "Loop data out"=w42:T5)  [unwired: 6 in]
  n10 = Select(t=T23."Disabled and Grayed Out" ("f"), s=w53, f=T23."Enabled") -> (s? t:f=w82:T23)
  n11 = property on="Measure" class="Bool"(error in=w83, "DisabledEnum"=w82) -> (error out=w43:errorcluster)  [unwired: 1 in, 1 out]
  n12 = Unbundle By Name("Session properties") -> ("Binary"=w27:bool)
  n13 = Unbundle By Name("IV measurement") -> ("Folder"=w5:path, "Name"=w45:string, "IV properties.Vstart"=w64:dbl[unit], "IV properties.Vstop"=w63:dbl[unit], "IV properties.Vpoints"=w65:dbl, "IV properties.Settling"=w18:dbl[unit], "IV properties.I limit"=w19:dbl[unit], "IV properties.Log mapping"=w41:bool, "IV properties.Averaging"=w10:dbl, "Time"=w25:timestamp, "IV properties.T"=w57:dbl[unit])
  n14 = Select(t="IV.bin", s=w27, f="IV.dat") -> (s? t:f=w60:string)
  n15 = local write "Folder"(w5) -> ()
  n16 = property on="Start voltage" class="DigNum (strict)"("Val(Sgnl)"=w64) -> (error out=w14:errorcluster)  [unwired: 2 in, 1 out]
  n17 = property on="Voltage points" class="DigNum (strict)"("Val(Sgnl)"=w65) -> (error out=w15:errorcluster)  [unwired: 2 in, 1 out]
  n18 = property on="Current limit" class="DigNum (strict)"("Val(Sgnl)"=w19) -> (error out=w13:errorcluster)  [unwired: 2 in, 1 out]
  n19 = property on="Averaging" class="DigNum (strict)"("Val(Sgnl)"=w10) -> (error out=w9:errorcluster)  [unwired: 2 in, 1 out]
  n20 = Build Path(base path="Workspace", name or relative path=w5) -> (appended path=w75:path)
  n21 = Concatenate Strings("myDLTS I-V measurement: " ("string"), w45) -> (w46:string)
  n22 = Build Path(base path=w75, name or relative path=w60) -> (appended path=w74:path)
  n23 = property class="VI"("Front Panel.Title"=w46) -> (error out=w30:errorcluster)  [unwired: 2 in, 1 out]
  n24 = call <vilib>:"Check if File or Folder Exists.vi"("error in (no error)"=w43, "path"=w74) -> ("error out"=w72:errorcluster, "file or folder exists?"=w56:bool, "dup path"=w73:path)  [unwired: 7 in]
  n25 = case shown="True" w56 {
    tunnel: w25 -> [_ w97]
    tunnel: w57 -> [_ w95]
    tunnel: [_ w94] -> w55
    tunnel: [w91 w93] -> w54
    tunnel: w53 -> [w92 _]
    frame False {
      n26 = Select(t="Edit only mode", s=w92, f="Set parameters and ") -> (s? t:f=w91:string)
    }
    frame True {
      n27 = Not A Number/Path/Refnum?(number/path/refnum=w95) -> (NaN/Path/Refnum?=w96:bool)
      n28 = case shown="False" w96 {
        tunnel: w97 -> [w100 w105]
        tunnel: w95 -> [_ w102]
        tunnel: [w99 w104] -> w94
        tunnel: [w98 w103] -> w93
        frame True {
          n29 = Format Into String(format string="The measurement was taken on %T.", w100) -> (resulting string=w98:string, error out=w99:errorcluster)  [unwired: 2 in]
        }
        frame False {
          n30 = Format Into String(format string="The measurement was taken %T at %.3g.", w105, w102) -> (resulting string=w103:string, error out=w104:errorcluster)  [unwired: 2 in]
        }
      }
    }
  }
  n31 = case shown="False" w56 {
    tunnel: w27 -> [_ w125]
    tunnel: w73 -> [_ w124]
    tunnel: w72 -> [w109 w123]
    tunnel: [w110 w115] -> w37
    tunnel: ["Measure" ("Boolean Text.Text") "Remeasure" ("Boolean Text.Text")] -> w35
    tunnel: [FALSE TRUE] -> w28
    frame False {
      n32 = property on="I-V" class="XYGraph (strict)"(error in=w109, "Value"=cluster{"2D data":dbl[], "2D data":dbl[]} {"2D data"=[], "2D data"=[]} ("I-V")) -> (error out=w108:errorcluster)  [unwired: 1 in, 1 out]
      n33 = invoke on="I-V Graph" class="XYGraph (strict)" method="Reinit To Default"(error in=w108) -> (error out=w110:errorcluster)  [unwired: 2 in, 2 out]
    }
    frame True {
      n34 = call "Read data file (SubVI).vi"("error in"=w123, "Binary"=w125, "file path in"=w124) -> ("error out"=w117:errorcluster, "2D data"=w122:dbl[][])  [unwired: 5 in, 2 out]
      n35 = Index Array(array=w122, index (col) #1=0 ("disabled index (col)"), index (col) #2=1 ("index (col)")) -> (element #1=w119:dbl[], element #2=w118:dbl[])  [unwired: 2 in]
      n36 = Bundle("2D data"=w119, "2D data"=w118) -> (w116:cluster{"2D data":dbl[], "2D data":dbl[]})  [unwired: 1 in]
      n37 = property on="I-V" class="XYGraph (strict)"(error in=w117, "Value"=w116) -> (error out=w115:errorcluster)  [unwired: 1 in, 1 out]
    }
  }
  n38 = property on="End voltage" class="DigNum (strict)"(error in=w14, "Val(Sgnl)"=w63) -> (error out=w62:errorcluster)  [unwired: 1 in, 1 out]
  n39 = property on="Settling" class="DigNum (strict)"(error in=w15, "Val(Sgnl)"=w18) -> (error out=w16:errorcluster)  [unwired: 1 in, 1 out]
  n40 = property on="Log mapping" class="Bool (strict)"(error in=w13, "Val(Sgnl)"=w41) -> (error out=w24:errorcluster)  [unwired: 1 in, 1 out]
  n41 = property on="Semi-log graph display" class="Bool (strict)"(error in=w9, "Val(Sgnl)"=FALSE ("Value (Signaling)")) -> (error out=w12:errorcluster)  [unwired: 1 in, 1 out]
  n42 = property on="Export" class="Bool"(error in=w30, "Visible"=w28) -> (error out=w29:errorcluster)  [unwired: 1 in, 1 out]
  n43 = property on="Measure" class="Bool"(error in=w37, "BoolText.Text"=w35) -> (error out=w36:errorcluster)  [unwired: 1 in, 1 out]
  n44 = property on="Measurement info" class="Str"(error in=w55, "Value"=w54) -> (error out=w40:errorcluster)  [unwired: 1 in, 1 out]
  n45 = Merge Errors(w36, w29, w62, w16, w24, w12, w40) -> (w8:errorcluster)
  n46 = disable-structure shown="Default" {
    disable-tunnel: w8 -> [w128 _]
    disable-tunnel: [w127 _] -> w7
    disable-tunnel: [w126 _] -> w6
    frame condition #0 (active) {
      n47 = call <vilib>:"Find Window.vi"("error in (no error)"=w128) -> ("error out"=w127:errorcluster, "Window Handle"=w126:refnum<k24>)  [unwired: 9 in]
    }
    frame condition #1 {
    }
  }
  n48 = Create User Event(user event datatype=w68, error in=w7) -> (user event=w48:refnum<user-event>, error out=w69:errorcluster)
  n49 = register-events(error in=w69, w48) -> (reference out=w70:refnum<event-registration>, error out=w71:errorcluster)  [unwired: 1 in]
  n50 = Generate Occurrence() -> (w1:refnum<k4>)
  n51 = Obtain Queue(name (unnamed)="Queue", element data type=cluster{"Data":variant, "Message":string} {"Data"=variant, "Message"=""}, error in (no error)=w71) -> (queue out=w49:refnum<queue>, error out=w76:errorcluster)  [unwired: 2 in, 1 out]
  n52 = while {
    shift-right: [w141] -> w79
    shift-left: w42 -> [w144]
    shift-right: [w142] -> w20
    shift-left: "IV measurement" -> [w143]
    shift-right: [w130] -> w52
    shift-left: w76 -> [w145]
    tunnel: w49 -> [w140]
    tunnel: w70 -> [w139]
    tunnel: [w138] -> w51
    shift-right: [w136] -> w38
    shift-left: FALSE -> [w137]
    tunnel: "Session properties" -> [w131]
    tunnel: w1 -> [w129]
    stop <- w146 stop-if-true
    w132 = T27 2 items=["no dialog", "OK message", "continue or stop message", "OK message + warnings", "continue/stop + warnings"] ("type of dialog (OK msg:1)")
    n53 = event shown="[12] \"Stop\": Value Change" {
      selector: w139 -> [_ _ _ _ _ _ _ _ _ _ _ _ _ _ _]
      dyn-events: [_ _ _ _ _ _ _ _ _ _ _ _ _ _ _] -> w138
      timeout: 1000 -> [_ _ _ _ _ _ _ _ _ _ _ _ _ _ _]
      tunnel: [_ _ FALSE TRUE _ _ _ _ _ _ _ _ _ _ _] -> w146
      tunnel: w145 -> [w152 w168 w173 w182 w192 w206 w211 w219 w230 w273 w280 w316 w334 w344 w377]
      tunnel: w144 -> [w151 w169 w178 w184 w189 w205 w213 w222 w235 w271 w275 w326 w339 w347 w380]
      tunnel: w143 -> [w153 w170 w179 w185 w190 w207 w214 w221 w234 w272 w276 w313 w338 w346 w373]
      tunnel: [w153 w170 w179 w185 w190 w207 w214 w221 w234 w272 w276 w311 w338 w341 w373] -> w142
      tunnel: [w151 w169 w178 w184 w189 w196 w213 w222 w235 w271 w275 w326 w339 w347 w380] -> w141
      tunnel: [w149 w168 w172 w182 w191 w197 w210 w219 w224 w273 w277 w297 w333 w340 w372] -> w134
      tunnel: w140 -> [_ _ w174 _ _ _ _ _ _ _ _ w321 _ _ _]
      tunnel: w137 -> [w148 w167 w171 w183 w188 w195 w212 w220 w248 w270 w274 _ w337 w345 w381]
      tunnel: [w148 w167 w171 w183 w188 w195 w212 w220 w248 w270 w274 TRUE w337 w342 w381] -> w136
      tunnel: w131 -> [_ _ _ _ _ _ _ _ w232 _ _ _ _ _ w374]
      tunnel: w129 -> [_ _ _ _ _ _ _ _ _ _ _ _ w336 _ _]
      event Timeout {
        n54 = event-data() -> ()  [unwired: 1 in, 3 out]
        n55 = Unbundle By Name(w151) -> ("Temp handle"=w147:T7, "Temp handle.Connected"=w150:bool)
        n56 = case shown="True" w150 {
          tunnel: w152 -> [w154 w159]
          tunnel: [w154 w161] -> w149
          tunnel: w147 -> [_ w157]
          frame False {
          }
          frame True {
            n57 = call "Temp ctrl - Read temp and stp.vi"("Error In"=w159, "Temp handle"=w157) -> ("Error Out"=w158:errorcluster, "Sample temperature"=→"Temperature":dbl[unit], "Setpoint"=w155:dbl[unit])  [unwired: 2 in, 2 out]
            n58 = property on="Setpoint" class="DigNum (strict)"(error in=w158) -> (error out=w162:errorcluster, "Key Focus"=w160:bool)  [unwired: 1 in, 1 out]
            n59 = case shown="False" w160 {
              tunnel: w162 -> [w164 w166]
              tunnel: [w165 w166] -> w161
              tunnel: w155 -> [w163 _]
              frame False {
                n60 = property on="Setpoint" class="DigNum (strict)"(error in=w164, "Value"=w163) -> (error out=w165:errorcluster)  [unwired: 1 in, 1 out]
              }
              frame True {
              }
            }
          }
        }
      }
      event Panel Resize {
        n61 = event-data() -> ()  [unwired: 1 in, 1 out]
      }
      event Panel Close? {
        n62 = event-data() -> ()  [unwired: 1 in, 1 out]
        n63 = Bundle By Name(cluster=cluster{"Data":variant, "Message":string} {"Data"=variant, "Message"=""}, "Message"="Stop") -> (w176:cluster{"Data":variant, "Message":string})
        n64 = Enqueue Element(queue=w174, element=w176, error in (no error)=w173) -> (error out=w172:errorcluster)  [unwired: 1 in, 2 out]
        n65 = event-data("Discard?"=TRUE) -> ()  [unwired: 1 in, 1 out]
      }
      event User Event {
        n66 = event-data() -> ()  [unwired: 1 in, 1 out]
      }
      event "Buttons.Help": Value Change {
        n67 = event-data() -> ()  [unwired: 1 in, 6 out]
        n68 = Unbundle By Name(w189) -> ("Paths.Manual"=w187:path)
        n69 = call "OpenDoc Browser.vi"("error in (no error)"=w192, "File"=w187) -> ("error out"=w191:errorcluster)  [unwired: 9 in]
      }
      event "Connect": Value Change {
        w203 = T23."Disabled and Grayed Out" ("f")
        w202 = T23."Enabled" ("Disabled")
        n70 = event-data() -> ()  [unwired: 1 in, 1 out]
        n71 = call "Connect devices (SubIV).vi"("Error In"=w206, "Devices"=T24 {"MFIA"=FALSE, "Temperature controller"=TRUE, "Source meter"=FALSE}, "Loop data in"=w205) -> ("Error Out"=w201:errorcluster, "Loop data out"=w196:T5)  [unwired: 6 in, 1 out]
        n72 = Unbundle By Name(w196) -> ("Temp handle.Connected"=w204:bool)
        n73 = Select(t=w202, s=w204, f=w203) -> (s? t:f=w199:T23)
        n74 = Select(t=w203, s=w204, f=w202) -> (s? t:f=w198:T23)
        n75 = property on="Setpoint" class="DigNum (strict)"(error in=w201, "DisabledEnum"=w199) -> (error out=w200:errorcluster)  [unwired: 1 in, 1 out]
        n76 = property on="Temperature" class="DigNum (strict)"(error in=w200, "DisabledEnum"=w199) -> (error out=w193:errorcluster)  [unwired: 1 in, 1 out]
        n77 = property on="Connect" class="Bool"(error in=w193, "DisabledEnum"=w198) -> (error out=w197:errorcluster)  [unwired: 1 in, 1 out]
      }
      event "Setpoint": Value Change {
        n78 = event-data() -> ()  [unwired: 1 in, 1 out]
        n79 = Unbundle By Name(w213) -> ("Temp handle"=w209:T7)
        n80 = call "Temp ctrl - Setpoint.vi"("Error In"=w211, "Setpoint"="Setpoint", "Temp handle"=w209) -> ("Error Out"=w210:errorcluster)  [unwired: 8 in]
      }
      event "Swap V": Value Change {
        n81 = event-data() -> ()  [unwired: 1 in, 1 out]
        n82 = local read "Start voltage"() -> (w217:dbl[unit])
        n83 = local read "End voltage"() -> (w218:dbl[unit])
        n84 = call "Synchronize Data Flow.vim"("input 4"=w217, "input 1"=w218) -> ("output 4"=w216:dbl[unit], "output 1"=w215:dbl[unit])  [unwired: 2 in, 2 out]
        n85 = local write "Start voltage"(w215) -> ()
        n86 = local write "End voltage"(w216) -> ()
      }
      event "Semi-log graph display": Value Change {
        n87 = event-data() -> ("NewVal"=w223:bool)  [unwired: 1 in]
        n88 = Unbundle By Name(w232) -> ("Binary"=w231:bool)
        n89 = local read "Workspace"() -> (w236:path)
        n90 = Unbundle By Name(w234) -> ("Folder"=w233:path)
        n91 = Build Path(base path=w236, name or relative path=w233) -> (appended path=w237:path)
        n92 = Select(t="IV.bin", s=w231, f="IV.dat") -> (s? t:f=w240:string)
        n93 = Build Path(base path=w237, name or relative path=w240) -> (appended path=w241:path)
        n94 = call <vilib>:"Check if File or Folder Exists.vi"("error in (no error)"=w230, "path"=w241) -> ("error out"=w229:errorcluster, "file or folder exists?"=w227:bool, "dup path"=w228:path)  [unwired: 7 in]
        n95 = case shown="True" w227 {
          tunnel: w231 -> [_ w259]
          tunnel: w229 -> [w249 w258]
          tunnel: w228 -> [_ w257]
          tunnel: [cluster{"2D data":dbl[], "2D data":dbl[]} {"2D data"=[], "2D data"=[]} w256] -> w226
          tunnel: [w249 w255] -> w225
          tunnel: w223 -> [_ w253]
          frame False {
          }
          frame True {
            n96 = call "Read data file (SubVI).vi"("error in"=w258, "Binary"=w259, "file path in"=w257) -> ("error out"=w255:errorcluster, "2D data"=w263:dbl[][])  [unwired: 5 in, 2 out]
            n97 = Index Array(array=w263, index (col) #1=0 ("disabled index (col)"), index (col) #2=1 ("index (col)")) -> (element #1=w260:dbl[], element #2=w251:dbl[])  [unwired: 2 in]
            n98 = Absolute Value(x=w251) -> (abs(x)=w252:dbl[])
            n99 = Select(t=w252, s=w253, f=w251) -> (s? t:f=w254:dbl[])
            n100 = Bundle("2D data"=w260, "2D data"=w254) -> (w256:cluster{"2D data":dbl[], "2D data":dbl[]})  [unwired: 1 in]
          }
        }
        n101 = Select(t=T25."Scientific" ("Y Scale.Display Format:Format"), s=w223, f=T25."SI" ("Y Scale.Display Format:Format")) -> (s? t:f=w242:T25)
        n102 = Select(t=enum8{"Linear", "Log"}."Log", s=w223, f=enum8{"Linear", "Log"}."Linear" ("Y Scale.Mapping Mode")) -> (s? t:f=w247:enum8{"Linear", "Log"})
        n103 = property on="I-V" class="XYGraph (strict)"(error in=w225, "YScale.Mapping Mode"=w247, "YScale.Format"=w242, "Value"=w226) -> (error out=w224:errorcluster)  [unwired: 1 in, 1 out]
      }
      event "Start voltage", "End voltage", "Voltage points": Value Change {
        n104 = event-data() -> ()  [unwired: 1 in, 1 out]
        n105 = local read "Voltage points"() -> (w267:dbl)
        n106 = local read "End voltage"() -> (w266:dbl[unit])
        n107 = local read "Start voltage"() -> (w265:dbl[unit])
        n108 = Subtract(x=w266, y=w265) -> (x-y=w269:dbl[unit])
        n109 = Decrement(x=w267) -> (x-1=w268:dbl)
        n110 = Divide(x=w269, y=w268) -> (x/y=→"Voltage step":dbl[unit])
      }
      event "Log mapping": Value Change {
        n111 = event-data() -> ("NewVal"=w279:bool)  [unwired: 1 in]
        n112 = Not(x=w279) -> (.not. x?=w278:bool)
        n113 = property on="Voltage step" class="DigNum (strict)"(error in=w280, "Visible"=w278) -> (error out=w277:errorcluster)  [unwired: 1 in, 1 out]
      }
      event "Measure": Value Change {
        # "Rename folder"
        # "New Folder"
        # "Old Folder"
        n114 = event-data() -> ()  [unwired: 1 in, 1 out]
        n115 = Unbundle By Name(w313) -> ("Folder"=w290:path, "IV properties"=w320:T2)
        n116 = Unbundle By Name(w326) -> ("Settings"=w325:T11)
        n117 = property on="Temperature" class="DigNum (strict)"(error in=w316) -> (error out=w301:errorcluster, "Value"=w309:dbl[unit])  [unwired: 1 in, 1 out]
        n118 = Bundle By Name(cluster=w320, "Vpoints"="Voltage points", "Vstart"="Start voltage", "Vstop"="End voltage", "I limit"="Current limit", "Settling"="Settling", "Log mapping"="Log mapping", "Averaging"="Averaging", "T"=w309) -> (w312:T2)
        n119 = property on="Export" class="Bool"(error in=w301, "Visible"=FALSE) -> (error out=w289:errorcluster)  [unwired: 1 in, 1 out]
        n120 = local read "Workspace"() -> (w291:path)
        n121 = call "myDLTS GUID.vi"() -> ("GUID"=w284:string)  [unwired: 1 in]
        n122 = Strip Path(path=w290) -> (stripped path=w295:path)  [unwired: 1 out]
        n123 = Build Path(base path=w295, name or relative path=w284) -> (appended path=w286:path)
        n124 = Build Path(base path=w291, name or relative path=w290) -> (appended path=w294:path)
        n125 = Get Date/Time In Seconds() -> (seconds since 1Jan1904=w285:timestamp)
        n126 = Build Path(base path=w291, name or relative path=w286) -> (appended path=w287:path)
        n127 = call <vilib>:"Check if File or Folder Exists.vi"("error in (no error)"=w289, "path"=w294) -> ("error out"=w293:errorcluster, "file or folder exists?"=w288:bool, "dup path"=w292:path)  [unwired: 7 in]
        n128 = local write "Folder"(w286) -> ()
        n129 = Bundle By Name(cluster=w313, "GUID"=w284, "Folder"=w286, "Time"=w285, "IV properties"=w312) -> (w311:T1)
        n130 = case shown="True" w288 {
          tunnel: w292 -> [_ w331]
          tunnel: w287 -> [_ w330]
          tunnel: w293 -> [w327 w329]
          tunnel: [w327 w328] -> w283
          frame False {
          }
          frame True {
            n131 = Move(source path=w331, error in=w329, 9:TRUE ("overwrite (F)"), 10:w330) -> (error out=w328:errorcluster)  [unwired: 1 in, 2 out]
          }
        }
        n132 = property on="Stop" class="Bool"(error in=w283, "DisabledEnum"=T23."Enabled" ("Disabled")) -> (error out=w282:errorcluster)  [unwired: 1 in, 1 out]
        n133 = Get Date/Time In Seconds() -> (seconds since 1Jan1904=w315:timestamp)
        n134 = Bundle By Name(cluster=cluster{"Settings":T11, "IV":T1} {"Settings"={"MFIA"={"Address"="", "Use compensation"=TRUE, "Shut down gracefully"=FALSE}, "Temp ctrl"={"Gain (P)"=0.0, "Reset (I)"=0.0, "Rate (D)"=0.0, "Stabilization rate"=0.0, "Stabilization delta"=0.0, "Type"=enum."Lake Shore 325", "Custom temp ctrl"={"VISA resource name"=""}, "Lakeshore 325"={"VISA name"="", "Loop"=0, "Heater Range"=1, "Heater Resistance"=0, "Sample sensor"=0, "Fast sensor"=0, "Slow sensor"=0}, "Lakeshore 331"={"VISA name"="", "Loop"=1, "Heater Range"=0, "Sample sensor"=0, "Fast sensor"=0, "Slow sensor"=0}, "Lakeshore 332"={"VISA name"="", "Loop"=1, "Heater Range"=0, "Sample sensor"=0, "Fast sensor"=0, "Slow sensor"=0}, "Lakeshore 335"={"VISA name"="", "Loop"=1, "Sample sensor"=0, "Fast sensor"=0, "Slow sensor"=0, "Heater Range"=0, "Output mode"=enum."Off"}, "Lakeshore 336"={"VISA name"="", "Loop"=1, "Output mode"=enum."Off", "Max current"=1.0, "Heater resistance"=1, "Sample sensor"=1, "Slow sensor"=1, "Fast sensor"=1}}, "Source-meter"={"Type"=enum."Custom", "Custom source-meter"={"VISA resource name"=""}, "Keithley 2600"={"VISA name"="", "Ignore ID Query"=FALSE, "SMU"=enum."Channel A"}, "Keithley 2400 Series"={"VISA name"="", "Ignore ID Query"=FALSE}}, "Other"={"Enable OriginLab"=FALSE, "Reader mode"=FALSE, "Auto-save"=FALSE}, "Defaults"={"IV properties"={"T"=0.0, "Vstart"=-0.5, "Vstop"=0.5, "Vpoints"=10.0, "Settling"=0.01, "I limit"=0.1, "Log mapping"=FALSE, "Averaging"=0.0}, "CV properties"={"T"=0.0, "Vstart"=-0.5, "Vstop"=0.5, "Vpoints"=10.0, "Precision"=enum."Normal", "Test signal"=0.01, "Auto I range"=FALSE, "Test frequency"=100000.0, "I range"=-2.0, "V range"=10.0, "Log mapping"=FALSE, "Rel perm"=0.0, "Area"=0.0, "Equivalent circuit model"=0}, "DLTS properties"={"Tstart"=0.0, "Instant start"=FALSE, "Tstop"=0.0, "T rate"=0.0, "Test signal"=0.0, "Test frequency"=0.0, "Bandwidth"=0.0, "Averaging"=0.0, "Vbias"=0.0, "Vpulse"=0.0, "pulse length"=0.0, "Pulse 2"=FALSE, "Vpulse 2"=0.0, "pulse length 2"=0.0, "I range"=-2.0, "V range"=10.0, "Emission rate"=[], "Sampling rate"=0.0, "Acq. delay"=0.0, "Filter order"=0, "Equivalent circuit model"=0}, "LDLTS properties"={"T"=0.0, "Test signal"=0.0, "Test frequency"=0.0, "Bandwidth"=0.0, "Averaging"=0.0, "Vbias"=0.0, "Vpulse"=0.0, "pulse length"=0.0, "Pulse 2"=FALSE, "Vpulse 2"=0.0, "pulse length 2"=0.0, "I range"=-2.0, "V range"=10.0, "Sampling rate"=0.0, "Acq. delay"=0.0, "Sampling time"=0.0, "Filter order"=0, "Equivalent circuit model"=0}}}, "IV"={"Name"="", "Comment"="", "Time"=timestamp(0 s since 1904-01-01), "Folder"=path "", "IV properties"={"T"=0.0, "Vstart"=-0.5, "Vstop"=0.5, "Vpoints"=10.0, "Settling"=0.01, "I limit"=0.1, "Log mapping"=FALSE, "Averaging"=0.0}, "GUID"=""}}, "Settings"=w325, "IV.IV properties"=w312, "IV.Time"=w315) -> (w322:cluster{"Settings":T11, "IV":T1})
        n135 = property on="Measure" class="Bool"(error in=w282, "DisabledEnum"=T23."Disabled and Grayed Out" ("Disabled")) -> (error out=w307:errorcluster)  [unwired: 1 in, 1 out]
        n136 = Bundle By Name(cluster=cluster{"Data":variant, "Message":string} {"Data"=variant, "Message"=""}, "Data"=w322, "Message"="Measure") -> (w323:cluster{"Data":variant, "Message":string})
        n137 = property on="Measurement info" class="Str"(error in=w307, "Value"="Wait" ("Measurement info")) -> (error out=w306:errorcluster)  [unwired: 1 in, 1 out]
        n138 = Enqueue Element(queue=w321, element=w323, error in (no error)=w306) -> (error out=w302:errorcluster)  [unwired: 1 in, 2 out]
        n139 = invoke on="I-V" class="XYGraph (strict)" method="Reinit To Default"(error in=w302) -> (error out=w297:errorcluster)  [unwired: 2 in, 2 out]
      }
      event "Stop": Value Change {
        n140 = event-data() -> ()  [unwired: 1 in, 1 out]
        n141 = Set Occurrence(w336) -> ()
        n142 = property on="Stop" class="Bool"(error in=w334, "DisabledEnum"=T23."Disabled and Grayed Out" ("Disabled")) -> (error out=w333:errorcluster)  [unwired: 1 in, 1 out]
      }
      event "Buttons.Information": Value Change {
        n143 = event-data() -> ("NewVal"=w343:bool)  [unwired: 1 in]
        n144 = case shown="True" w343 {
          tunnel: w346 -> [w349 w356]
          tunnel: w344 -> [w348 w359]
          tunnel: [w348 w357] -> w340
          tunnel: [w349 w355] -> w341
          tunnel: w345 -> [w350 w354]
          tunnel: [w350 w353] -> w342
          frame False {
          }
          frame True {
            n145 = Unbundle By Name(w356) -> ("Name"=w361:string, "Comment"=w360:string)
            n146 = call "Measurement renamer.vi"("error in (no error)"=w359, "Comment In"=w360, "Measurement name In"=w361) -> ("error out"=w357:errorcluster, "Canceled"=w358:bool, "Comment Out"=w351:string, "Measurement name Out"=w352:string)  [unwired: 1 in]
            n147 = case shown="False" w358 {
              tunnel: w356 -> [w365 w368]
              tunnel: [w364 w368] -> w355
              tunnel: w354 -> [_ w367]
              tunnel: [TRUE w367] -> w353
              tunnel: w352 -> [w363 _]
              tunnel: w351 -> [w362 _]
              frame False {
                n148 = Bundle By Name(cluster=w365, "Name"=w363, "Comment"=w362) -> (w364:T1)
              }
              frame True {
              }
            }
          }
        }
      }
      event "Buttons.Export": Value Change {
        n149 = event-data() -> ()  [unwired: 1 in, 1 out]
        n150 = Unbundle By Name(w380) -> ("Settings.Other.Enable OriginLab"=w378:bool)
        n151 = local read "Workspace"() -> (w375:path)
        n152 = Bundle By Name(cluster=T26 {"Clipboard"=TRUE, "dat"=TRUE, "iso"=FALSE, "Origin"=FALSE, "Excel"=FALSE} ("Available options"), "Origin"=w378) -> (w379:T26)
        n153 = call "Export dialog.vi"("error in (no error)"=w377, "Available options"=w379) -> ("error out"=w371:errorcluster, "Option"=w376:T28)  [unwired: 7 in, 1 out]
        n154 = case shown="\"Clipboard\"" w376 {
          tunnel: w375 -> [_ w385 w390 w396]
          tunnel: w374 -> [_ _ _ w395]
          tunnel: w373 -> [_ w384 w389 w394]
          tunnel: [w382 w387 w388 w393] -> w372
          tunnel: w371 -> [w382 w386 w391 w392]
          tunnel: "myDLTS file path" -> [_ w383 _ _]
          frame "Canceled", Default {
          }
          frame "Dat" {
            n155 = call-poly "Export single dat - cluster.vi"(".myDLTS file path"=w383, "Error In"=w386, "Workspace"=w385, "IV measurement"=w384) -> ("Error Out"=w387:errorcluster)  [unwired: 4 in]
          }
          frame "Clipboard" {
            n156 = call-poly "Export single clipboard - cluster.vi"("Error In"=w391, "Workspace"=w390, "IV measurement"=w389) -> ("Error Out"=w388:errorcluster)  [unwired: 5 in]
          }
          frame "Origin" {
            n157 = call-poly "Export Origin.vi"("Error In"=w392, "Workspace"=w396, "Session properties"=w395, "IV measurement"=w394) -> ("Error Out"=w393:errorcluster)  [unwired: 7 in]
          }
        }
      }
    }
    n158 = call <vilib>:"General Error Handler.vi"("type of dialog (OK msg:1)"=w132, "error in (no error)"=w134) -> ("error out"=w133:errorcluster)  [unwired: 9 in, 4 out]
    n159 = call <vilib>:"Clear Errors.vi"("error in (no error)"=w133) -> ("error out"=w130:errorcluster)  [unwired: 5 in, 1 out]
  }
  "Loop data out" <- w79
  "Modified" <- w38
  "IV measurement out" <- w20
  n160 = while {
    tunnel: w49 -> [w411]
    shift-right: [w399] -> w31
    shift-left: w76 -> [w412]
    tunnel: w48 -> [w406]
    tunnel: w42 -> [w404]
    tunnel: "Session properties" -> [w400]
    tunnel: w6 -> [w398]
    tunnel: w1 -> [w397]
    stop <- w405 stop-if-true
    w401 = T27 2 items=["no dialog", "OK message", "continue or stop message", "OK message + warnings", "continue/stop + warnings"] ("type of dialog (OK msg:1)")
    n161 = Dequeue Element(queue=w411, error in (no error)=w412) -> (element=w410:cluster{"Data":variant, "Message":string}, error out=w407:errorcluster)  [unwired: 1 in, 2 out]
    n162 = Unbundle(w410) -> ("Data"=w408:variant, "Message"=w409:string)
    n163 = case shown="\"Measure\"" w409 {
      tunnel: w408 -> [_ w455 _]
      tunnel: w407 -> [w413 w456 w470]
      tunnel: w406 -> [_ _ w469]
      tunnel: [w413 w425 w467] -> w403
      tunnel: [_ _ TRUE] -> w405
      tunnel: w404 -> [_ w454 _]
      tunnel: w400 -> [_ w443 _]
      tunnel: w398 -> [_ w423 _]
      tunnel: w397 -> [_ w417 _]
      frame "", Default {
      }
      frame "Measure" {
        w421 = T29 0 items=["NoProgress"=0, "Indeterminate"=1, "Normal"=2, "Error"=4, "Paused"=8] ("State (No Progress)")
        # "Save data"
        # "Absolute value of I if semi-log scale is on"
        # "Perform IV sweep"
        n164 = Variant To Data(error in=w456, type=cluster{"Settings":T11, "IV":T1} {"Settings"={"MFIA"={"Address"="", "Use compensation"=TRUE, "Shut down gracefully"=FALSE}, "Temp ctrl"={"Gain (P)"=0.0, "Reset (I)"=0.0, "Rate (D)"=0.0, "Stabilization rate"=0.0, "Stabilization delta"=0.0, "Type"=enum."Lake Shore 325", "Custom temp ctrl"={"VISA resource name"=""}, "Lakeshore 325"={"VISA name"="", "Loop"=0, "Heater Range"=1, "Heater Resistance"=0, "Sample sensor"=0, "Fast sensor"=0, "Slow sensor"=0}, "Lakeshore 331"={"VISA name"="", "Loop"=1, "Heater Range"=0, "Sample sensor"=0, "Fast sensor"=0, "Slow sensor"=0}, "Lakeshore 332"={"VISA name"="", "Loop"=1, "Heater Range"=0, "Sample sensor"=0, "Fast sensor"=0, "Slow sensor"=0}, "Lakeshore 335"={"VISA name"="", "Loop"=1, "Sample sensor"=0, "Fast sensor"=0, "Slow sensor"=0, "Heater Range"=0, "Output mode"=enum."Off"}, "Lakeshore 336"={"VISA name"="", "Loop"=1, "Output mode"=enum."Off", "Max current"=1.0, "Heater resistance"=1, "Sample sensor"=1, "Slow sensor"=1, "Fast sensor"=1}}, "Source-meter"={"Type"=enum."Custom", "Custom source-meter"={"VISA resource name"=""}, "Keithley 2600"={"VISA name"="", "Ignore ID Query"=FALSE, "SMU"=enum."Channel A"}, "Keithley 2400 Series"={"VISA name"="", "Ignore ID Query"=FALSE}}, "Other"={"Enable OriginLab"=FALSE, "Reader mode"=FALSE, "Auto-save"=FALSE}, "Defaults"={"IV properties"={"T"=0.0, "Vstart"=-0.5, "Vstop"=0.5, "Vpoints"=10.0, "Settling"=0.01, "I limit"=0.1, "Log mapping"=FALSE, "Averaging"=0.0}, "CV properties"={"T"=0.0, "Vstart"=-0.5, "Vstop"=0.5, "Vpoints"=10.0, "Precision"=enum."Normal", "Test signal"=0.01, "Auto I range"=FALSE, "Test frequency"=100000.0, "I range"=-2.0, "V range"=10.0, "Log mapping"=FALSE, "Rel perm"=0.0, "Area"=0.0, "Equivalent circuit model"=0}, "DLTS properties"={"Tstart"=0.0, "Instant start"=FALSE, "Tstop"=0.0, "T rate"=0.0, "Test signal"=0.0, "Test frequency"=0.0, "Bandwidth"=0.0, "Averaging"=0.0, "Vbias"=0.0, "Vpulse"=0.0, "pulse length"=0.0, "Pulse 2"=FALSE, "Vpulse 2"=0.0, "pulse length 2"=0.0, "I range"=-2.0, "V range"=10.0, "Emission rate"=[], "Sampling rate"=0.0, "Acq. delay"=0.0, "Filter order"=0, "Equivalent circuit model"=0}, "LDLTS properties"={"T"=0.0, "Test signal"=0.0, "Test frequency"=0.0, "Bandwidth"=0.0, "Averaging"=0.0, "Vbias"=0.0, "Vpulse"=0.0, "pulse length"=0.0, "Pulse 2"=FALSE, "Vpulse 2"=0.0, "pulse length 2"=0.0, "I range"=-2.0, "V range"=10.0, "Sampling rate"=0.0, "Acq. delay"=0.0, "Sampling time"=0.0, "Filter order"=0, "Equivalent circuit model"=0}}}, "IV"={"Name"="", "Comment"="", "Time"=timestamp(0 s since 1904-01-01), "Folder"=path "", "IV properties"={"T"=0.0, "Vstart"=-0.5, "Vstop"=0.5, "Vpoints"=10.0, "Settling"=0.01, "I limit"=0.1, "Log mapping"=FALSE, "Averaging"=0.0}, "GUID"=""}}, Variant=w455) -> (data=w427:cluster{"Settings":T11, "IV":T1}, error out=w424:errorcluster)
        n165 = disable-structure shown="TARGET_TYPE==Windows" {
          disable-tunnel: w424 -> [w464 _]
          disable-tunnel: w423 -> [w463 w465]
          disable-tunnel: [w461 w465] -> w422
          frame condition #0 (active) {
            w462 = T29 1 items=["NoProgress"=0, "Indeterminate"=1, "Normal"=2, "Error"=4, "Paused"=8] ("State (No Progress)")
            n166 = call <vilib>:"Set Progress State.vi"("error in (no error)"=w464, "State (No Progress)"=w462, "Window Handle"=w463) -> ("dup Window Handle"=w461:refnum<k24>)  [unwired: 7 in, 1 out]
          }
          frame condition #1 {
          }
        }
        n167 = Unbundle By Name(w443) -> ("Binary"=w442:bool)
        n168 = Unbundle By Name(w454) -> ("Source-meter handle"=w436:T22)
        n169 = Unbundle By Name(w427) -> ("IV.IV properties"=w435:T2)
        n170 = control-ref of="I-V"() -> (w418:refnum<vi>)
        n171 = control-ref of="Measurement info"() -> (w419:refnum<vi>)
        n172 = call "Source-meter - IV sweep.vi"("XY Graph to update"=w418, "String reference"=w419, "Error In"=w424, "Stop occurrence"=w417, "IV properties"=w435, "Source-meter handle"=w436) -> ("error out"=w428:errorcluster, "Voltage (V)"=w434:dbl[], "Current (A)"=w432:dbl[])  [unwired: 3 in]
        n173 = local read "Semi-log graph display"() -> (w431:bool)
        n174 = Absolute Value(x=w432) -> (abs(x)=w433:dbl[])
        n175 = Select(t=w433, s=w431, f=w432) -> (s? t:f=w430:dbl[])
        n176 = Bundle("Voltage (V)"=w434, "Current (A)"=w430) -> (→"I-V":T30)  [unwired: 1 in]
        n177 = Build Array(w434, w432) -> (w448:dbl[][])
        n178 = Transpose 2D Array(2D array=w448) -> (transposed array=w447:dbl[][])
        n179 = local read "Workspace"() -> (w449:path)
        n180 = Select(t="IV.bin", s=w442, f="IV.dat") -> (s? t:f=w452:string)
        n181 = Build Path(base path=w449, name or relative path="Folder") -> (appended path=w453:path)
        n182 = Build Path(base path=w453, name or relative path=w452) -> (appended path=w446:path)
        n183 = call "Write data file (SubVI).vi"("error in"=w428, "Binary"=w442, "2D data"=w447, "file path in"=w446) -> ("error out"=w438:errorcluster)  [unwired: 6 in, 1 out]
        n184 = property on="Export" class="Bool"(error in=w438, "Visible"=TRUE) -> (error out=w441:errorcluster)  [unwired: 1 in, 1 out]
        n185 = property on="Measure" class="Bool"(error in=w441, "BoolText.Text"="Remeasure" ("Boolean Text.Text"), "DisabledEnum"=T23."Enabled" ("Disabled")) -> (error out=w415:errorcluster)  [unwired: 1 in, 1 out]
        n186 = property on="Stop" class="Bool"(error in=w415, "DisabledEnum"=T23."Disabled and Grayed Out" ("Disabled")) -> (error out=w414:errorcluster)  [unwired: 1 in, 1 out]
        n187 = property on="Measurement info" class="Str"(error in=w414, "Val(Sgnl)"="Done!" ("Value (Signaling)")) -> (error out=w426:errorcluster)  [unwired: 1 in, 1 out]
        n188 = disable-structure shown="TARGET_TYPE==Windows" {
          disable-tunnel: w426 -> [w460 _]
          disable-tunnel: [w459 _] -> w425
          disable-tunnel: w422 -> [w458 _]
          disable-tunnel: w421 -> [w457 _]
          frame condition #0 (active) {
            n189 = call <vilib>:"Set Progress State.vi"("error in (no error)"=w460, "State (No Progress)"=w457, "Window Handle"=w458) -> ("error out"=w459:errorcluster)  [unwired: 7 in, 1 out]
          }
          frame condition #1 {
          }
        }
      }
      frame "Stop" {
        n190 = Generate User Event(user event=w469, event data cluster=TRUE ("event data"), error in=w470) -> (error out=w467:errorcluster)  [unwired: 1 in, 1 out]
      }
    }
    n191 = call <vilib>:"General Error Handler.vi"("type of dialog (OK msg:1)"=w401, "error in (no error)"=w403) -> ("error out"=w402:errorcluster)  [unwired: 9 in, 4 out]
    n192 = call <vilib>:"Clear Errors.vi"("error in (no error)"=w402) -> ("error out"=w399:errorcluster)  [unwired: 5 in, 1 out]
  }
  n193 = Unregister For Events(event registration refnum=w51, error in=w52) -> (error out=w11:errorcluster)
  n194 = Destroy User Event(user event=w48, error in=w11) -> (error out=w33:errorcluster)
  n195 = Merge Errors(w33, w31) -> (w32:errorcluster)
  n196 = Release Queue(queue=w49, error in (no error)=w32) -> (error out=→"Error Out":errorcluster)  [unwired: 1 in, 2 out]
